vi "信号光谱9 - BN-BN.vi"() -> ()   [LabVIEW 2018]
uses:
  <vilib>/Utility/NIReport.llb/Report Type.ctl
  <vilib>/Utility/file.llb/Write Delimited Spreadsheet (DBL).vi
  <vilib>/Instr/_visa.llb/VISA Configure Serial Port (Instr).vi
  <vilib>/addons/_office/excel.llb/Excel Get Data ([str]).vi
  <vilib>/Utility/NIReport.llb/NI_report.lvclass
  <vilib>/Analysis/NI_AALBase.lvlib
  <vilib>/ptbypt/NI_PtbyPt.lvlib
  <vilib>/Utility/NIReport.llb/NI_ReportGenerationCore.lvlib
  <vilib>/addons/_office/NI_ReportGenerationToolkit.lvlib
  <vilib>/Utility/NIReport.llb/Excel/NI_Excel.lvclass
panel:
  out "数值":i32
  in  "停止预测":bool
  in  "误差值":dbl=0.5
  out "target angle":dbl
  out "图片地址 2":string
  out "图片地址 3":string
  out "原始峰值":dbl
  out "拟合峰值":dbl
  in  "角度倍乘系数":dbl=1.5
  out "结果展示":dbl[][](array[numeric])=[[37.33100777239877, 2672.955043835526, 29.54153292599307, 222755.0, 50.0], [37.36593979472361, 2672.656498058864, 30.113284142729572, 222833.0, 50.0], [38.96986225690859, 2673.3337152325566, 33.38805102415213, 222910.0, 75.0], [37.39946104045098, 2676.4005085744548, 31.215565446104666, 222948.0, 47.0], [35.862209164247574, 2671.7826876859012, 30.355582265151796, 223028.0, 47.0]]
  out "Δw2>C":bool=TRUE
  out "Δw1>C":bool=TRUE
  out "θi":dbl
  in  "w0":dbl format="%#_13g"
  in  "C=w-w0":dbl=180.0 format="%#_13g"
  in  "上升下降沿/s":dbl format="%.2p"
  in  "延时/s":dbl format="%.2p"
  in  "占空比/%":dbl=3.0 format="%.2p"
  in  "高电平/V":dbl=4.0 format="%.2p"
  in  "频率/Hz":dbl=6000.0 format="%.3p"
  in  "低电平/V":dbl min=0.0 max=5.0 format="%.2p"
  in  "Enable":bool
  in  "上升下降沿":i32(ring)=1 items=["上升沿", "下降沿"]
  in  "输出信号波形":u16(ring) items=["Pulse"]
  out "Output":bool
  in  "VISA 信号发生器":refnum<visa-resource-name>="USB0::0x1AB1::0x0641::DG4E192200870::INSTR"
  out "Output 2":bool
  in  "Enable 2":bool
  in  "上升下降沿/s 2":dbl format="%.2p"
  in  "延时/s 2":dbl format="%.2p"
  in  "占空比/% 2":dbl=3.0 format="%.2p"
  in  "高电平/V 2":dbl=0.002 format="%.2p"
  in  "频率/Hz 2":dbl=6000.0 format="%.3p"
  in  "低电平/V 2":dbl min=0.0 max=5.0 format="%.2p"
  in  "上升下降沿 2":i32(ring)=1 items=["上升沿", "下降沿"]
  in  "输出信号波形 2":u16(ring) items=["Pulse"]
  in  "终止测量":bool
  in  "测量次数":i32=1
  out "best fit":cluster{"Y":dbl[], "Y":dbl[]}[](graph)
  in  "拟合终点":i32=850
  in  "拟合起点":i32=200
  out "current angle":dbl
  out "图片地址":string
  in  "开光时间/ms":u32=50
  out "最终存储路径 2":path
  out "照明光error out":errorcluster
  in  "照明光":bool
  in  "stop bits (10: 1 bit)":u16(ring)=10 items=["1.0"=10, "1.5"=15, "2.0"=20]
  in  "parity (0:none)":enum16{"None", "Odd", "Even", "Mark", "Space"}(ring)
  in  "data bits (8)":u16=8 min=5 max=8 step=1
  in  "baud rate":u32=9600 caption="baud rate (115200)" min=9600 max=115200
  in  "照明光VISA":refnum<visa-resource-name>="COM12"
  out "正在测量":bool
  in  "滤波阈值":dbl=3000.0 format="%#_13g"
  out "范围内？":bool[](array[boolean])
  out "w":dbl
  out "xc":dbl
  out "拟合参数":dbl[](array[numeric])
  out "最终存储路径":path
  in  "停止程序":bool
  out "configure error out":errorcluster
  in  "设置参数":bool
  out "output control error  4":errorcluster
  in  "低电平持续输出":bool
  out "output control error  5":errorcluster
  out "output control error":errorcluster
  in  "开始测量":bool
  in  "channel输出口":i32(ring) items=["Channel 1", "Channel 2"]
  out "output control error":errorcluster
  out "Spectrum":cluster{"Y":dbl[], "Y":dbl[]}[](graph)
  out "波长范围":dbl[](array[numeric])
  in  "?":enum32{"IHR 550", "CCD"}(tab)
  in  "Move To\nTarget Positions":bool
  out "Current UniqueID":string="Mono4"
  in  "Mono ID":string(combo)="Mono1"
  in  "Connect":bool
  out "Initialized JY":bool=TRUE
  in  "Force\nInitialization":bool
  in  "Target Grating":string(combo)="2"
  out "Current Description":string="1" caption="Description"
  out "Grating Index":i32=1
  out "Current Grating":dbl=1200.0
  out "Units":string="nm"
  out "Current WL":dbl=897.9988
  out "Exit Mirror\nPosition":i32(ring)=2 items=["EntranceMirror", "ExitMirror", "Front", "Side"]
  out "Entrance Mirror\nPosition":i32(ring)=2 items=["EntranceMirror", "ExitMirror", "Front", "Side"]
  out "Units 2":string="mm"
  out "Front Entrance":dbl
  in  "Target WL":dbl=516.0
  in  "Exit Mirror":u16(ring)=3 caption="Target Position Exit Mirror" items=["Front"=2, "Side"=3]
  in  "Entrance Mirror":u16(ring)=2 caption="Target Position\nEntrance Mirror" items=["Front"=2, "Side"=3]
  in  "Target\nFront Entrance":dbl=2.0
  in  "Commande tab":T1(tab)
  in  "Area Number to Display":i32
  in  "Reformat":bool
  in  "GAIN":u16(ring)=2 caption="Device Name" items=["High Light", "Best Dynamic Range", "High Sensitivity"]
  in  "ADC":u16(ring) caption="Device Name" items=["20 kHz       ", " 1 MHz       ", " 1 MHz Ultra "]
  in  "Number of Areas :":u16=1 min=1 step=1
  in  "Integration time (ms) :":i16=10000
  out "Uniques ID":u16(ring) items=["CCD1", "CCD2"]
  in  "Device Name":u16(ring) items=["Synapse CCD (Lateral)", "Synapse_IGA (Axial)"]
  in  "Signal type :":enum16{"TTL Rising Edge", "TTL Falling Edge"}(ring)=enum."TTL Falling Edge"
  in  "Trigger Type :":u16(ring) items=["On Start"=1, "Per Acquisition"=2]
  in  "trigSigTypeString":string
  in  "trigEventString":string
  in  "Enable InputTriggers :":bool
  in  "Number of Cleans":i32=1
  in  "MultiAcqShutterMode":i32(ring)=3 items=["Open For All Spectra"=1, "Open for Each Spectrum"=3]
  in  "Accumulations:":u16=10 min=1 step=1
  in  "Multi Accumulation mode:":bool
  out "Y Pixels:":i32=256
  out "DataSize":i32=1024
  out "X Pixels:":i32=1024
  out "Firmware\nVersion":string="V1.20 CCD_4000"
  out "initialized ?":bool=TRUE
  in  "Continuous":bool
  in  "CCD Busy":bool
  out "indicator":string="Ready !"
  in  "initialize":bool
  in  "ShutterOpen":bool=TRUE caption="Shutter enable"
  in  "Acquire":bool
  in  "Temperature":bool
  in  "Setup":bool
  out "Acq Time(ms)":u32=3401
  in  "Save Backlight":bool
  in  "cut backlight":bool
  out "backlight":bool=TRUE
  in  "是否拟合":bool
  in  "是否保存":bool
  in  "Close":bool=TRUE
  out "JYCCDLib.IJYCCDReqd":refnum<k7>
  out "areas :":i32[][](array[numeric])=[[1], [1], [1], [1024], [256], [1], [256]]
  in  "Constante de condition\n(Voir l'aide contextuelle)":bool
  out "temp graph":dbl(graph)=-134.538067
  out "ADC Number":i32[](array[numeric])=[0, 1, 2, 3, 4]
  out "Gain Number":i32[](array[numeric])=[10, 11, 12, 13, 8, 2]
  out "trigAddress":i32
  out "Data":i32[][](graph)
  out "error out":errorcluster
  out "Gratings":dbl[](array[numeric])=[1200.0, 300.0]
  out "Backlight":i32[][](graph)
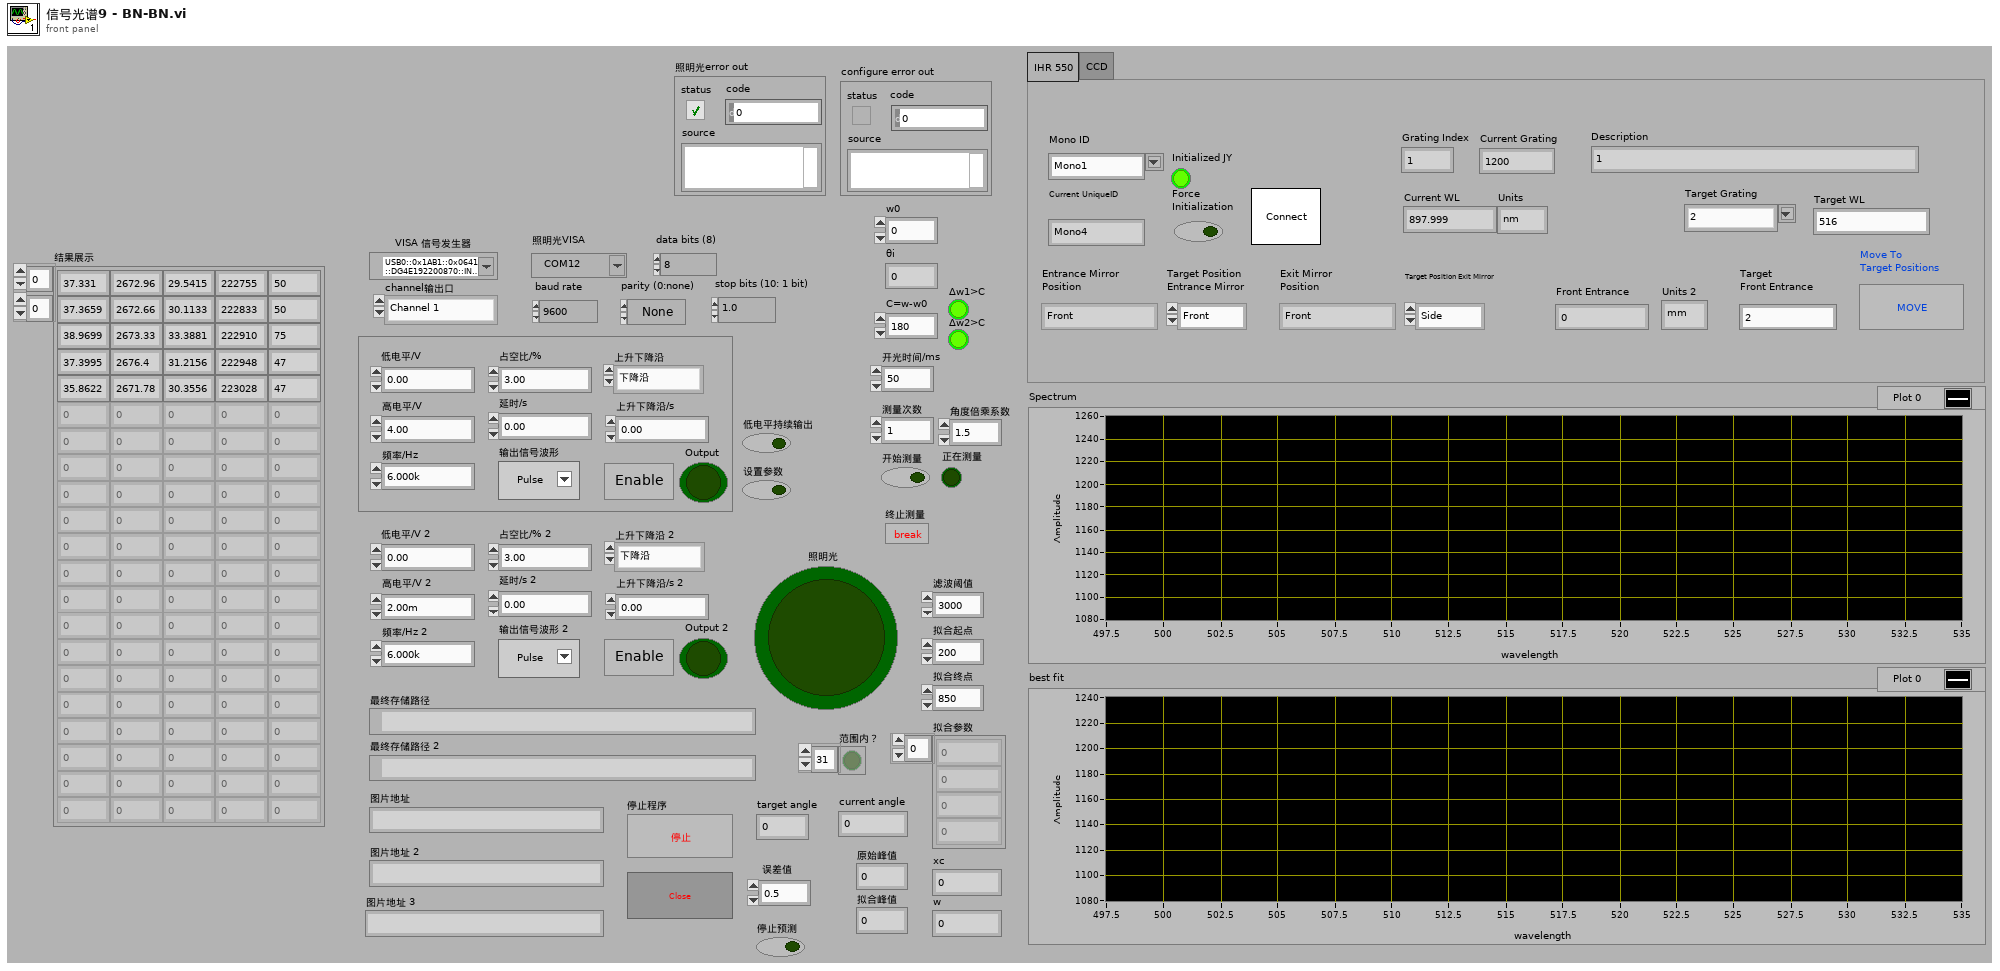
[diagram p1: front panel]
types:
  T1 = enum32{"Settings", "Trigger In", "Multi-Accu.", "Infos"}
  T2 = enum8{"Enabled", "Disabled", "Disabled and Grayed Out"}
  T3 = enum16{"maximized", "minimized", "normal", "no change"}
  T4 = typedef "NI_ReportGenerationCore.lvlib/Report Type.ctl" = enum16{"HTML", "Word", "Excel"}
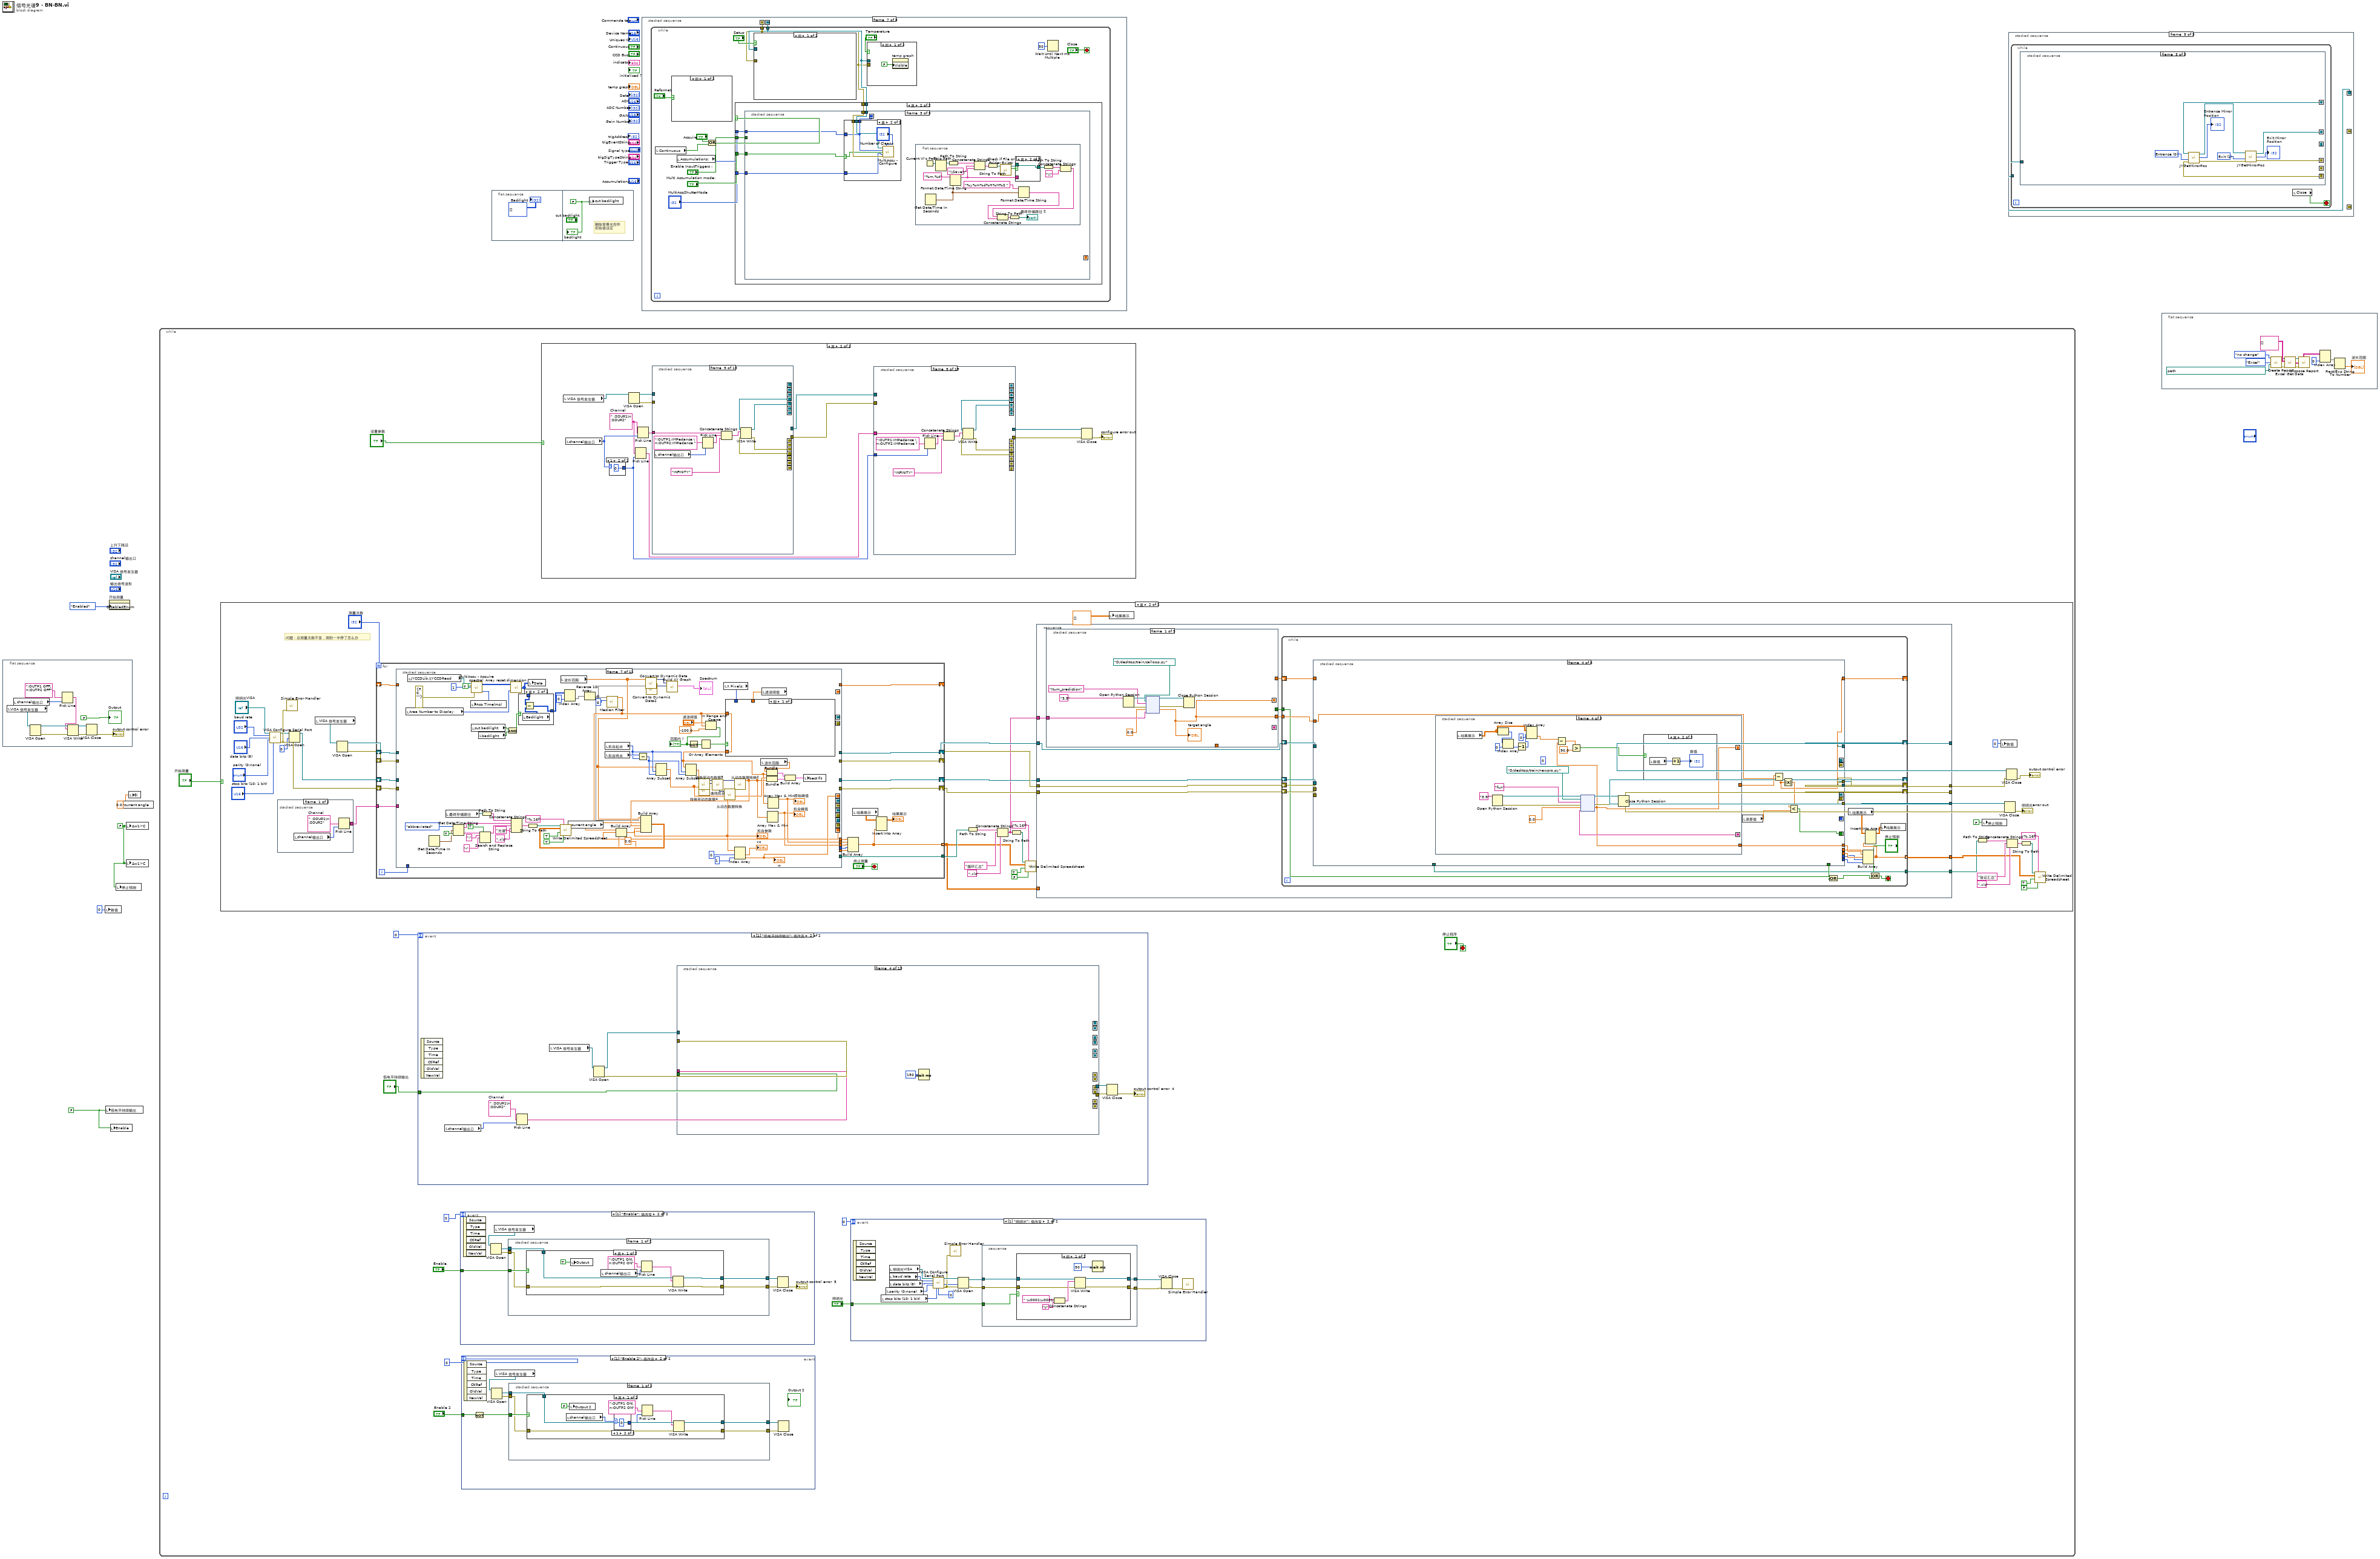
[diagram p0: block diagram]
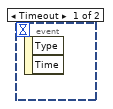
[diagram p2: hidden frame]
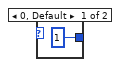
[diagram p3: hidden frame]
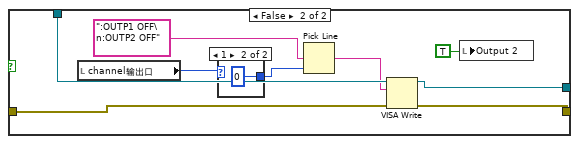
[diagram p4: hidden frame]
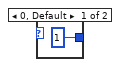
[diagram p5: hidden frame]
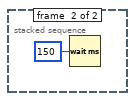
[diagram p6: hidden frame]
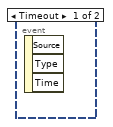
[diagram p7: hidden frame]
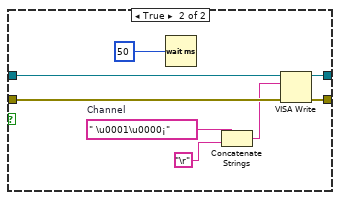
[diagram p8: hidden frame]
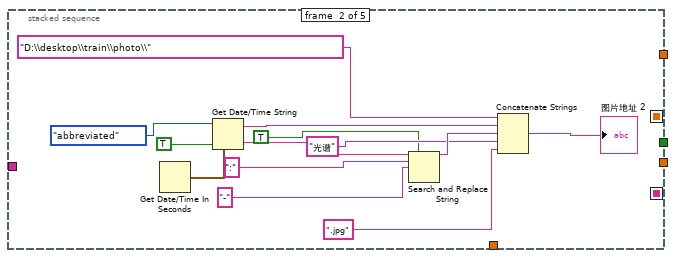
[diagram p10: hidden frame]
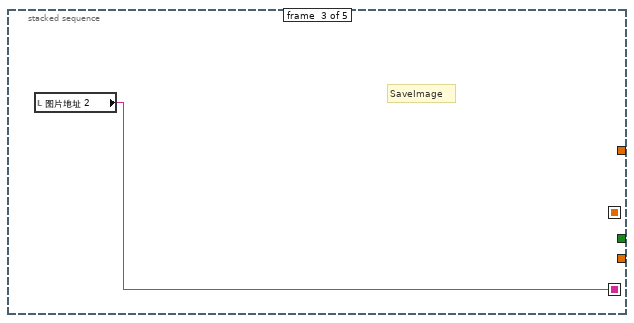
[diagram p11: hidden frame]
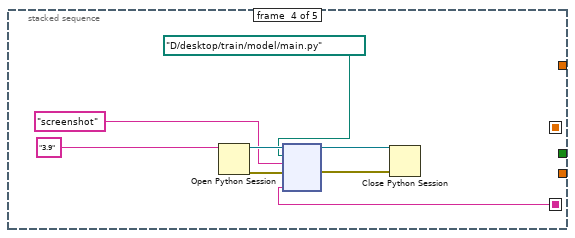
[diagram p12: hidden frame]
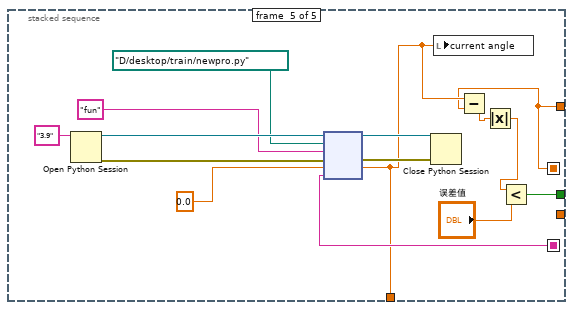
[diagram p13: hidden frame]
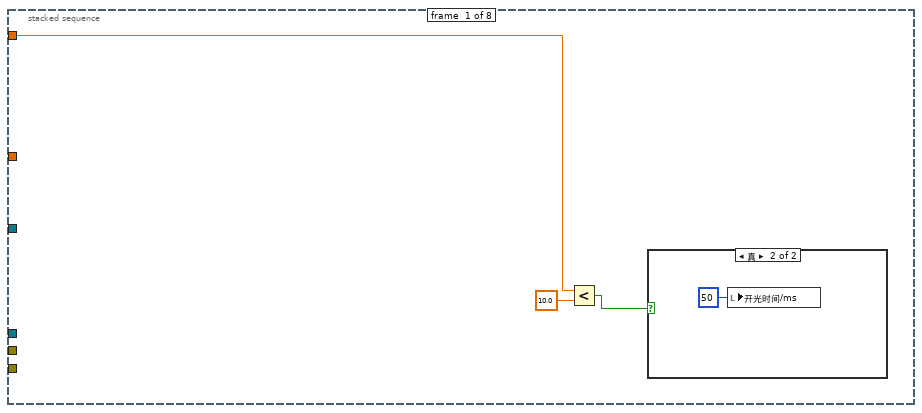
[diagram p14: hidden frame]
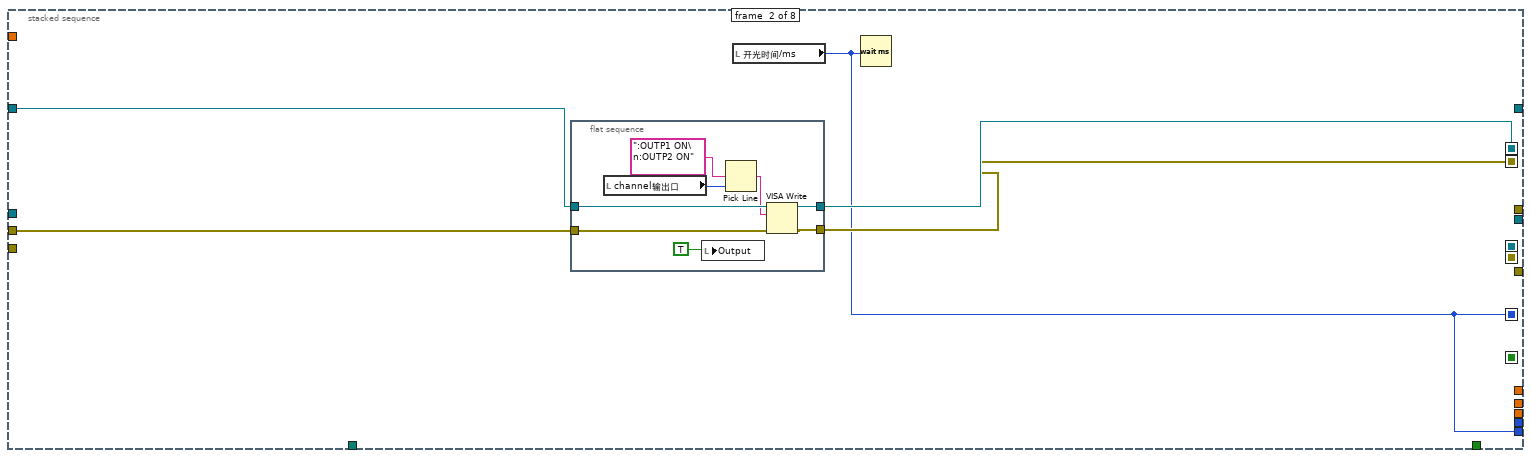
[diagram p16: hidden frame]
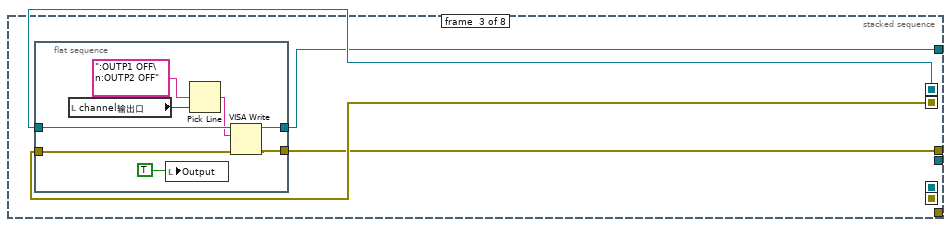
[diagram p17: hidden frame]
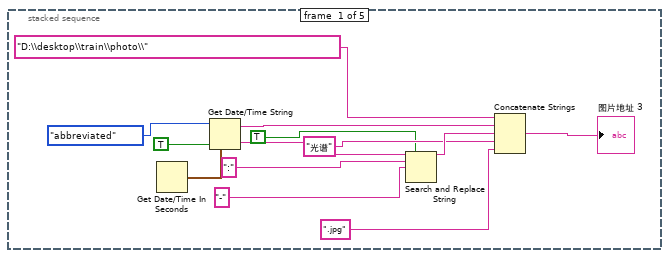
[diagram p18: hidden frame]
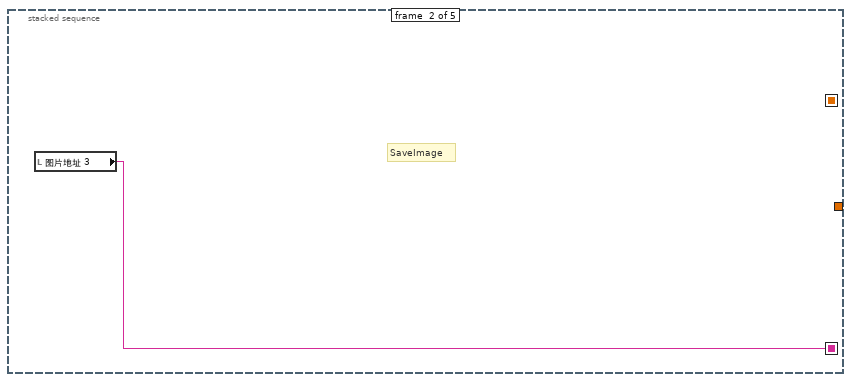
[diagram p19: hidden frame]
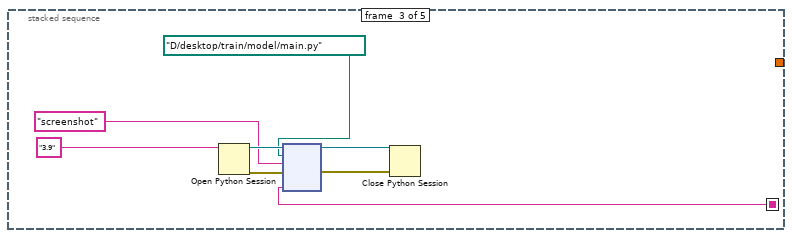
[diagram p20: hidden frame]
diagram:
  w2 = FALSE ("Δw1>C")
  w3 = 0.0 ("angle")
  w4 = FALSE
  n1 = flat-sequence {
    frame #0 {
      n2 = local read "VISA 信号发生器"() -> (w9:refnum<visa-resource-name>)
      n3 = local read "channel输出口"() -> (w7:i32)
      n4 = VISA Open(VISA resource name=w9) -> (VISA resource name=w15:refnum<visa-resource-name>, error out=w14:errorcluster)  [unwired: 4 in]
      n5 = Pick Line(multi-line string=":OUTP1 OFF\n:OUTP2 OFF" ("write buffer"), line index=w7) -> (output string=w6:string)  [unwired: 1 in]
      n6 = VISA Write(VISA resource name=w15, write buffer=w6, error in (no error)=w14) -> (VISA resource name out=w12:refnum<visa-resource-name>, error out=w11:errorcluster)  [unwired: 1 out]
      n7 = VISA Close(VISA resource name=w12, error in (no error)=w11) -> (error out=→"output control error":errorcluster)
      "Output" <- FALSE ("布尔")
    }
  }
  n8 = local write "数值"(0 ("数值")) -> ()
  n9 = local write "低电平持续输出"(w4) -> ()
  n10 = property on="开始测量" class="Bool"("DisabledEnum"=T2."Enabled" ("禁用")) -> ()  [unwired: 2 in, 2 out]
  n11 = local write "Enable"(w4) -> ()
  n12 = local write "停止预测"(w2) -> ()
  n13 = local write "current angle"(w3) -> ()
  n14 = local write "Δw1>C"(w2) -> ()
  n15 = local write "Δw1>C"(w2) -> ()
  n16 = local write "θi"(w3) -> ()
  n17 = while {
    stop <- "停止程序" stop-if-true
    n18 = case shown="真" "开始测量" {
      frame False {
      }
      frame True {
        # "问题：总测量次数不变，测到一半停了怎么办"
        n19 = call-poly "VISA Configure Serial Port"("VISA resource name"="照明光VISA", "baud rate (9600)"="baud rate", "data bits (8)"="data bits (8)", "parity (0:none)"="parity (0:none)", "stop bits (10: 1 bit)"="stop bits (10: 1 bit)") -> ("VISA resource name out"=w139:refnum<visa-resource-name>, "error out"=w140:errorcluster)  [unwired: 9 in]
        n20 = stacked-sequence {
          tunnel: [w437 _] -> w141
          frame #0 {
            w438 = " :SOUR1\n :SOUR2"  # Channel
            n21 = local read "channel输出口"() -> (w439:i32)
            n22 = Pick Line(multi-line string=w438, line index=w439) -> (output string=w437:string)  [unwired: 1 in]
          }
          frame #1 {
            w440 = FALSE ("Δw1>C")
            n23 = local write "Δw1>C"(w440) -> ()
            n24 = local write "Δw2>C"(w440) -> ()
          }
        }
        n25 = call <vilib>:"Simple Error Handler.vi"("error in (no error)"=w140) -> ()  [unwired: 4 in, 5 out]
        n26 = VISA Open(access mode=0, error in (no error)=w140, VISA resource name=w139) -> (VISA resource name=w132:refnum<visa-resource-name>, error out=w131:errorcluster)  [unwired: 2 in]
        n27 = local read "VISA 信号发生器"() -> (w144:refnum<visa-resource-name>)
        n28 = VISA Open(VISA resource name=w144) -> (VISA resource name=w143:refnum<visa-resource-name>, error out=w142:errorcluster)  [unwired: 4 in]
        n29 = for {
          N: "测量次数" -> [_]
          tunnel: w141 -> [w460]
          shift-right: [w456] -> w119
          shift-left: w143 -> [w462]
          shift-right: [w455] -> w118
          shift-left: w142 -> [w461]
          shift-right: [w454] -> w113
          shift-left: w132 -> [w459]
          shift-right: [w453] -> w112
          shift-left: w131 -> [w458]
          tunnel: [w443] -> w120 mode=indexing
          shift-right: [w448] -> _
          shift-left: _ -> [w447]
          tunnel: [w444] -> w122
          i -> [w446]
          stop <- "终止测量" stop-if-true
          n30 = stacked-sequence {
            seq-local: [w469 _ _ _ _ _ _ _ _ _ _ _] -> [_ w489 _ _ _ _ _ _ _ _ _ _]
            seq-local: [w468 _ _ _ _ _ _ _ _ _ _ _] -> [_ w488 _ _ _ _ _ _ _ _ _ _]
            seq-local: [_ _ _ _ _ w574 _ _ _ _ _ _] -> [_ _ _ _ _ _ _ _ w692 _ _ _]
            seq-local: [_ _ _ _ _ w573 _ _ _ _ _ _] -> [_ _ _ _ _ _ _ _ w695 _ _ _]
            seq-local: [_ w487 _ _ _ _ _ _ _ _ _ _] -> [_ _ _ _ w560 _ _ _ _ _ _ _]
            seq-local: [_ w486 _ _ _ _ _ _ _ _ _ _] -> [_ _ _ _ w559 _ _ _ _ _ _ _]
            seq-local: [_ _ _ _ w558 _ _ _ _ _ _ _] -> [_ _ _ _ _ _ _ w678 _ _ _ _]
            seq-local: [_ _ _ _ w557 _ _ _ _ _ _ _] -> [_ _ _ _ _ _ _ w677 _ _ _ _]
            seq-local: [_ _ w498 _ _ _ _ _ _ _ _ _] -> [_ _ _ _ _ _ _ _ _ _ w704 _]
            seq-local: [_ _ _ _ _ _ w589 _ _ _ _ _] -> [_ _ _ _ _ _ _ _ _ _ w699 _]
            seq-local: [w463 _ _ _ _ _ _ _ _ _ _ _] -> [_ _ _ _ _ _ w587 _ _ _ _ _]
            tunnel: w462 -> [w471 _ _ _ _ _ _ _ _ _ _ _]
            tunnel: w461 -> [w470 _ _ _ _ _ _ _ _ _ _ _]
            tunnel: [_ _ _ _ _ _ _ w676 _ _ _ _] -> w456
            tunnel: [_ _ _ _ _ _ _ w675 _ _ _ _] -> w455
            tunnel: w460 -> [_ _ _ _ _ _ _ _ _ _ _ _]
            tunnel: w459 -> [_ _ _ _ _ w577 _ _ _ _ _ _]
            tunnel: w458 -> [_ _ _ _ _ w576 _ _ _ _ _ _]
            tunnel: [_ _ _ _ _ _ _ _ w694 _ _ _] -> w454
            tunnel: [_ _ _ _ _ _ _ _ w693 _ _ _] -> w453
            tunnel: [_ _ w498 _ _ _ _ _ _ _ _ _] -> w452
            tunnel: [_ _ _ _ _ _ w584 _ _ _ _ _] -> w451
            tunnel: [_ _ _ _ _ _ w583 _ _ _ _ _] -> w450
            tunnel: [_ _ _ w532 _ _ _ _ _ _ _ _] -> w449
            tunnel: [w463 _ _ _ _ _ _ _ _ _ _ _] -> w445
            tunnel: [_ _ w498 _ _ _ _ _ _ _ _ _] -> w448
            tunnel: w447 -> [_ _ _ _ _ _ _ _ _ _ w703 _]
            tunnel: w446 -> [_ _ _ _ _ _ _ _ _ _ w701 _]
            tunnel: [_ _ _ w531 _ _ _ _ _ _ _ _] -> w444
            frame #0 {
              n31 = Wait Until Next ms Multiple(millisecond multiple=u32 1 ("毫秒倍数")) -> ()  [unwired: 1 out]
              n32 = flat-sequence {
                tunnel: w471 -> [w485]
                tunnel: w470 -> [w484]
                tunnel: [w479] -> w469
                tunnel: [w478] -> w468
                frame #0 {
                  n33 = local read "channel输出口"() -> (w481:i32)
                  n34 = local write "Output"(TRUE ("布尔")) -> ()
                  n35 = Pick Line(multi-line string=":OUTP1 ON\n:OUTP2 ON" ("write buffer"), line index=w481) -> (output string=w480:string)  [unwired: 1 in]
                  n36 = VISA Write(VISA resource name=w485, write buffer=w480, error in (no error)=w484) -> (VISA resource name out=w479:refnum<visa-resource-name>, error out=w478:errorcluster)  [unwired: 1 out]
                }
              }
              n37 = local read "Δw1>C"() -> (w465:bool)
              n38 = local read "Δw2>C"() -> (w466:bool)
              n39 = And(x=w465, y=w466) -> (x .and. y?=w464:bool)
              n40 = case shown="真" w464 {
                tunnel: [w474 w475] -> w463
                tunnel: "开光时间/ms" -> [w474 w477]
                frame False {
                }
                frame True {
                  n41 = Divide(x=w477, y=u32 4) -> (x/y=w475:dbl)
                }
              }
              n42 = Wait (ms)(milliseconds to wait=w463) -> ()  [unwired: 1 out]
              "正在测量" <- TRUE
            }
            frame #1 {
              n43 = flat-sequence {
                tunnel: w489 -> [w497]
                tunnel: w488 -> [w496]
                tunnel: [w491] -> w487
                tunnel: [w490] -> w486
                frame #0 {
                  n44 = local read "channel输出口"() -> (w493:i32)
                  n45 = local write "Output"(FALSE ("布尔")) -> ()
                  n46 = Pick Line(multi-line string=":OUTP1 OFF\n:OUTP2 OFF" ("write buffer"), line index=w493) -> (output string=w492:string)  [unwired: 1 in]
                  n47 = VISA Write(VISA resource name=w497, write buffer=w492, error in (no error)=w496) -> (VISA resource name out=w491:refnum<visa-resource-name>, error out=w490:errorcluster)  [unwired: 1 out]
                }
              }
            }
            frame #2 {
              n48 = stacked-sequence {
                seq-local: [_ w512 _ _] -> [_ _ w513 w522]
                tunnel: [_ _ _ w521] -> w498
                frame #0 {
                  n49 = Get Date/Time In Seconds() -> (seconds since 1Jan1904=w508:timestamp)
                  n50 = Get Date/Time String(date format (0)=enum16{"short", "long", "abbreviated"}."abbreviated" ("日期格式(0)"), seconds (now)=w508, want seconds? (F)=TRUE ("需要秒？(F)")) -> (date string=w511:string, time string=w509:string)
                  n51 = Search and Replace String(replace all?=TRUE ("替换全部？(F)"), input string=w509, search string=":" ("搜索字符串"), replace string="-" ("替换字符串(\"\")")) -> (result string=w510:string)  [unwired: 4 in, 3 out]
                  n52 = Concatenate Strings("D:\\desktop\\train\\photo\\", w511, w510, "光谱" ("字符串"), ".jpg" ("字符串")) -> (→"图片地址":string)
                }
                frame #1 {
                  # "SaveImage"
                  n53 = local read "图片地址"() -> (w512:string)
                }
                frame #2 {
                  n54 = Open Python Session(python version="3.9" ("Python version")) -> (session out=w520:refnum<k35>, error out=w518:errorcluster)  [unwired: 2 in]
                  n55 = node(w520, path "D:/desktop/train/model/main.py" ("module path"), "screenshot" ("function name"), w518, w513) -> (w519:refnum<k35>, w517:errorcluster)  [unwired: 3 in, 2 out]
                  n56 = Close Python Session(session in=w519, error in=w517) -> ()  [unwired: 1 out]
                }
                frame #3 {
                  n57 = Open Python Session(python version="3.9" ("Python version")) -> (session out=w529:refnum<k35>, error out=w527:errorcluster)  [unwired: 2 in]
                  n58 = node(w529, path "D:/desktop/train/newpro.py" ("module path"), "fun" ("function name"), w527, 0.0, w522) -> (w528:refnum<k35>, w526:errorcluster, w521:dbl)  [unwired: 1 in, 2 out]
                  "current angle" <- w521
                  n59 = Close Python Session(session in=w528, error in=w526) -> ()  [unwired: 1 out]
                }
              }
            }
            frame #3 {
              n60 = Current VI's Path() -> (path=w541:path)
              n61 = Get Date/Time In Seconds() -> (seconds since 1Jan1904=w534:timestamp)
              n62 = Strip Path(path=w541) -> (stripped path=w542:path)  [unwired: 1 out]
              n63 = Path To String(path=w542) -> (string=w543:string)
              n64 = Format Date/Time String(time format string (%c)="%m-%d" ("时间格式字符串(%c)"), seconds (now)=w534) -> (date/time string=w549:string)  [unwired: 1 in]
              n65 = Concatenate Strings(w543, "\\Save\\" ("字符串"), w549) -> (w544:string)
              n66 = String To Path(string=w544) -> (path=w545:path)
              n67 = call <vilib>:"Check if File or Folder Exists.vi"("path"=w545) -> ("file or folder exists?"=w546:bool, "dup path"=w548:path)  [unwired: 8 in, 1 out]
              n68 = case shown="真" w546 {
                tunnel: [w555 w556] -> w547
                tunnel: w548 -> [w554 w556]
                tunnel: w549 -> [w553 _]
                frame False {
                  n69 = Create Folder(prompt (Create Folder)=w553, path (use dialog)=w554) -> (created path=w555:path)  [unwired: 1 in, 2 out]
                }
                frame True {
                }
              }
              n70 = Format Date/Time String(time format string (%c)="%y%m%d%H%M%S" ("时间格式字符串(%c)"), seconds (now)=w534) -> (date/time string=w552:string)  [unwired: 1 in]
              n71 = Path To String(path=w547) -> (string=w550:string)
              n72 = Concatenate Strings(w550, "\\" ("字符串")) -> (w551:string)
              n73 = Format Date/Time String(time format string (%c)="%H%M%S" ("时间格式字符串(%c)"), seconds (now)=w534) -> (date/time string=w533:string)  [unwired: 1 in]
              n74 = Concatenate Strings(w551, w552) -> (w540:string)
              n75 = String To Path(string=w540) -> (path=w531:path)
              "最终存储路径" <- w531
              n76 = Decimal String To Number(string=w533) -> (number=w532:i32)  [unwired: 2 in, 1 out]
            }
            frame #4 {
              n77 = flat-sequence {
                tunnel: w560 -> [w569]
                tunnel: w559 -> [w568]
                tunnel: [w564] -> w558
                tunnel: [w563] -> w557
                frame #0 {
                  n78 = local read "channel输出口"() -> (w562:i32)
                  n79 = case shown="1" w562 {
                    tunnel: [1 0] -> w561
                    frame 0, Default {
                    }
                    frame 1 {
                    }
                  }
                  n80 = local write "Output 2"(FALSE ("布尔")) -> ()
                  n81 = Pick Line(multi-line string=":OUTP1 OFF\n:OUTP2 OFF" ("write buffer"), line index=w561) -> (output string=w565:string)  [unwired: 1 in]
                  n82 = VISA Write(VISA resource name=w569, write buffer=w565, error in (no error)=w568) -> (VISA resource name out=w564:refnum<visa-resource-name>, error out=w563:errorcluster)  [unwired: 1 out]
                }
              }
            }
            frame #5 {
              w572 = " \u0001\u0001¢"  # Channel
              n83 = Wait (ms)(milliseconds to wait=500) -> ()  [unwired: 1 out]
              n84 = Concatenate Strings(w572, "\r") -> (w578:string)
              n85 = local write "照明光"(FALSE ("照明光")) -> ()
              n86 = VISA Write(VISA resource name=w577, write buffer=w578, error in (no error)=w576) -> (VISA resource name out=w574:refnum<visa-resource-name>, error out=w573:errorcluster)  [unwired: 1 out]
            }
            frame #6 {
              n87 = local read "Area Number to Display"() -> (w628:i32)
              n88 = local read "JYCCDLib.IJYCCDReqd"() -> (w624:refnum<k7>)
              n89 = Get Date/Time In Seconds() -> (seconds since 1Jan1904=w637:timestamp)
              n90 = local read "最终存储路径"() -> (w651:path)
              n91 = Get Date/Time String(date format (0)=enum16{"short", "long", "abbreviated"}."abbreviated" ("日期格式(0)"), seconds (now)=w637, want seconds? (F)=TRUE ("需要秒？(F)")) -> (date string=w645:string, time string=w640:string)
              n92 = call "MultiAccu - Acquire spectral.vi"("error in"=errorcluster {"status"=FALSE, "code"=0, "source"=""}, "Accumulations:"=u16 1, "ShutterOpen"=TRUE, "JYCCDLib.IJYCCDReqd"=w624) -> ("Acq Time(ms)"=w630:u32, "Array Out"=w629:i32[][][])  [unwired: 1 out]
              n93 = local write "Acq Time(ms)"(w630) -> ()
              n94 = local read "cut backlight"() -> (w612:bool)
              n95 = local read "backlight"() -> (w610:bool)
              n96 = Search and Replace String(replace all?=TRUE ("替换全部？(F)"), input string=w640, search string=":" ("搜索字符串"), replace string="-" ("替换字符串(\"\")")) -> (result string=w644:string)  [unwired: 4 in, 3 out]
              n97 = Path To String(path=w651) -> (string=w634:string)
              n98 = And(x=w612, y=w610) -> (x .and. y?=w611:bool)
              n99 = call "Array reset dimension.vi"("Area Number"=w628, "Array In"=w629) -> ("Array Out"=w614:i32[][])
              n100 = Concatenate Strings(w634, w645, w644, "光谱" ("字符串"), ".xls" ("字符串")) -> (w649:string)
              n101 = case shown="真" w611 {
                tunnel: [w671 w673] -> w613
                tunnel: w614 -> [w671 w672]
                frame False {
                }
                frame True {
                  n102 = local read "Backlight"() -> (w674:i32[][])
                  n103 = Subtract(x=w672, y=w674) -> (x-y=w673:i32[][])
                }
              }
              n104 = String To Path(string=w649) -> (path=w650:path)
              n105 = local write "Data"(w614) -> ()
              n106 = local read "波长范围"() -> (w582:dbl[])
              n107 = Index Array(array=w613, index (row)=0 ("索引 (行)")) -> (element=w652:i32[])  [unwired: 1 in]
              n108 = local read "current angle"() -> (w593:dbl)
              n109 = Reverse 1D Array(array=w652) -> (reversed array=w581:i32[])
              n110 = local read "拟合起点"() -> (w600:i32)
              n111 = local read "拟合终点"() -> (w602:i32)
              n112 = call <vilib>:"Median Filter.vi"("left rank"=6, "X"=w581) -> ("Filtered X"=w591:dbl[])  [unwired: 8 in, 1 out]
              n113 = Build Array(w593, w587, 0.0 ("元素")) -> (w592:dbl[])
              n114 = Subtract(x=w602, y=w600) -> (x-y=w599:i32)
              n115 = call "Convert to Dynamic Data"("Array"=w582) -> ("Dynamic Data Type"=w621:dynamicdata)  [unwired: 3 in]
              n116 = call "Convert to Dynamic Data2"("Array"=w581) -> ("Dynamic Data Type"=w620:dynamicdata)  [unwired: 3 in]
              n117 = Array Subset(array=w582, index=w600, length=w599) -> (w598:dbl[])
              n118 = call "Build XY Graph"("Y Input"=w620, "X Input"=w621) -> ("XY Graph"=→"Spectrum":cluster{"Y":dbl[], "Y":dbl[]}[])  [unwired: 8 in, 1 out]
              n119 = call "转换至动态数据4"("Array"=w598) -> ("Dynamic Data Type"=w618:dynamicdata)  [unwired: 3 in]
              n120 = In Range and Coerce(upper limit="滤波阈值", x=w591, lower limit=-100.0) -> (In Range?=w605:bool[])  [unwired: 1 out]
              "范围内？" <- w605
              n121 = Not(x=w605) -> (.not. x?=w604:bool[])
              n122 = Or Array Elements(Boolean array=w604) -> (logical OR=w607:bool)
              n123 = local read "X Pixels:"() -> (w606:i32)
              n124 = local read "波长范围"() -> (w594:dbl[])
              n125 = local read "滤波阈值"() -> (w603:dbl)
              n126 = case shown="假" w607 {
                tunnel: w606 -> [_ w658]
                tunnel: w591 -> [w654 w657]
                tunnel: [w654 w656] -> w585
                tunnel: w603 -> [_ w655]
                frame False {
                }
                frame True {
                  n127 = for {
                    N: w658 -> [_]
                    tunnel: w657 -> [w662] mode=indexing
                    tunnel: [w661] -> w656 mode=indexing
                    shift-right: [w661] -> _
                    shift-left: _ -> [w660]
                    tunnel: w655 -> [w659]
                    n128 = Greater?(x=w662, y=w659) -> (0:w664:bool)
                    n129 = Less?(x=w662, y=-100.0) -> (x < y?=w665:bool)
                    n130 = Or(x=w664, y=w665) -> (x .or. y?=w663:bool)
                    n131 = case shown="真" w663 {
                      tunnel: w662 -> [w667 _]
                      tunnel: [w667 w669] -> w661
                      tunnel: w660 -> [_ w670]
                      frame False {
                      }
                      frame True {
                        n132 = call <vilib>:"Median Filter PtByPt.vi"("rank"=5, "x"=w670) -> ("Filtered x"=w669:dbl)  [unwired: 2 in, 1 out]
                      }
                    }
                  }
                }
              }
              n133 = Array Subset(array=w585, index=w600, length=w599) -> (w601:dbl[])
              n134 = call "转换至动态数据3"("Array"=w601) -> ("Dynamic Data Type"=w619:dynamicdata)  [unwired: 3 in]
              n135 = call "曲线拟合"("Locations"=w618, "Signals"=w619) -> ("best fit"=w623:dynamicdata, "non-linear coefficients"=w622:dynamicdata)  [unwired: 5 in, 3 out]
              n136 = call "从动态数据转换"("Dynamic Data Type"=w622) -> ("Array"=w615:dbl[])  [unwired: 3 in]
              "拟合参数" <- w615
              n137 = call "从动态数据转换2"("Dynamic Data Type"=w623) -> ("Array"=w586:dbl[])  [unwired: 3 in]
              n138 = Build Array(w582, w581, w591, w586, w615, w592) -> (w653:dbl[][])
              n139 = call-poly <vilib>:"Write Delimited Spreadsheet.vi"("file path (dialog if empty)"=w650, "format (%.3f)"="%.16f", "2D data"=w653, "append to file? (new file:F)"=TRUE ("append to file? (F)"), "transpose? (no:F)"=TRUE ("transpose? (F)")) -> ()  [unwired: 9 in, 2 out]
              n140 = Index Array(array=w615, index #1=0 ("索引"), index #2=1 ("索引")) -> (element #1=→"xc":dbl, element #2=w589:dbl)
              "w" <- w589
              n141 = Bundle("波长范围"=w594, "Filtered X"=w585) -> (w597:cluster{"波长范围 ":dbl[], "Filtered X":dbl[]})  [unwired: 1 in]
              n142 = Bundle(w598, "Array"=w586) -> (w596:cluster{dbl[], "Array":dbl[]})  [unwired: 1 in]
              n143 = Array Max & Min(array=w586) -> (max value=w583:dbl)  [unwired: 3 out]
              "拟合峰值" <- w583
              n144 = Array Max & Min(array=w585) -> (max value=w584:dbl)  [unwired: 3 out]
              "原始峰值" <- w584
              n145 = Build Array(w597, w596) -> (w595:cluster{"波长范围 ":dbl[], "Array":dbl[]}[])
              n146 = local write "best fit"(w595) -> ()
            }
            frame #7 {
              n147 = flat-sequence {
                tunnel: w678 -> [w687]
                tunnel: w677 -> [w686]
                tunnel: [w682] -> w676
                tunnel: [w681] -> w675
                frame #0 {
                  n148 = local read "channel输出口"() -> (w680:i32)
                  n149 = case shown="1" w680 {
                    tunnel: [1 0] -> w679
                    frame 0, Default {
                    }
                    frame 1 {
                    }
                  }
                  n150 = local write "Output 2"(TRUE ("布尔")) -> ()
                  n151 = Pick Line(multi-line string=":OUTP1 ON\n:OUTP2 ON" ("write buffer"), line index=w679) -> (output string=w683:string)  [unwired: 1 in]
                  n152 = VISA Write(VISA resource name=w687, write buffer=w683, error in (no error)=w686) -> (VISA resource name out=w682:refnum<visa-resource-name>, error out=w681:errorcluster)  [unwired: 1 out]
                }
              }
            }
            frame #8 {
              w690 = " \u0001\u0000¡"  # Channel
              n153 = Concatenate Strings(w690, "\r") -> (w696:string)
              n154 = VISA Write(VISA resource name=w692, write buffer=w696, error in (no error)=w695) -> (VISA resource name out=w694:refnum<visa-resource-name>, error out=w693:errorcluster)  [unwired: 1 out]
              n155 = local write "照明光"(TRUE ("照明光")) -> ()
            }
            frame #9 {
              n156 = Wait (ms)(milliseconds to wait=1200) -> ()  [unwired: 1 out]
            }
            frame #10 {
              n157 = Greater Or Equal?(x=w701, y=1) -> (x >= y?=w702:bool)
              n158 = case shown="真" w702 {
                tunnel: w704 -> [_ w710]
                tunnel: w703 -> [_ w711]
                tunnel: w699 -> [w705 w712]
                frame False {
                  n159 = local write "w0"(w705) -> ()
                }
                frame True {
                  n160 = local read "Δw1>C"() -> (w709:bool)
                  n161 = case shown="假" w709 {
                    tunnel: w712 -> [w731 w751]
                    tunnel: w711 -> [w721 _]
                    tunnel: w710 -> [w722 _]
                    frame False {
                      # "判断Δw突变位置并记录当前θ值"
                      # "根据θ变化速度改变开光时间"
                      n162 = local read "w0"() -> (w729:dbl)
                      n163 = Subtract(x=w722, y=w721) -> (x-y=w724:dbl)
                      n164 = local read "开光时间/ms"() -> (w727:u32)
                      n165 = Subtract(x=w729, y=w731) -> (x-y=w734:dbl)
                      n166 = Absolute Value(x=w724) -> (abs(x)=w726:dbl)
                      n167 = Absolute Value(x=w734) -> (abs(x)=w732:dbl)
                      n168 = Greater Or Equal?(x=w726, y=4.0) -> (x >= y?=w725:bool)
                      n169 = Greater Or Equal?(x=w732, y="C=w-w0") -> (x >= y?=w730:bool)
                      n170 = case shown="真" w730 {
                        tunnel: w721 -> [_ w749]
                        frame False {
                          w747 = FALSE ("Δw1>C")
                          n171 = local write "Δw1>C"(w747) -> ()
                          n172 = local write "Δw2>C"(w747) -> ()
                        }
                        frame True {
                          "θi" <- w749
                          "Δw1>C" <- TRUE ("布尔")
                        }
                      }
                      n173 = case shown="假" w725 {
                        tunnel: w726 -> [w739 _]
                        tunnel: w727 -> [w736 w746]
                        tunnel: [w735 w744] -> w728
                        frame False {
                          n174 = Less Or Equal?(x=w739, y=1.0) -> (x <= y?=w737:bool)
                          n175 = case shown="假" w737 {
                            tunnel: w736 -> [w740 w743]
                            tunnel: [w740 w742] -> w735
                            frame False {
                            }
                            frame True {
                              n176 = Multiply(x=w743, y="角度倍乘系数") -> (x*y=w742:dbl)
                            }
                          }
                        }
                        frame True {
                          n177 = Divide(x=w746, y=1.6) -> (x/y=w744:dbl)
                        }
                      }
                      n178 = local write "开光时间/ms"(w728) -> ()
                    }
                    frame True {
                      # "再次判断Δw，排除坏点影响"
                      n179 = local read "Δw2>C"() -> (w750:bool)
                      n180 = case shown="假" w750 {
                        tunnel: w751 -> [w756 _]
                        frame False {
                          n181 = local read "C=w-w0"() -> (w753:dbl)
                          n182 = local read "w0"() -> (w757:dbl)
                          n183 = Subtract(x=w757, y=w756) -> (x-y=w759:dbl)
                          n184 = Absolute Value(x=w759) -> (abs(x)=w758:dbl)
                          n185 = Add(x=w753, y=0.5) -> (x+y=w752:dbl)
                          n186 = Greater Or Equal?(x=w758, y=w752) -> (x >= y?=w755:bool)
                          n187 = case shown="真" w755 {
                            frame False {
                              n188 = local write "θi"(0.0 ("θi")) -> ()
                              n189 = local write "Δw1>C"(FALSE ("Δw1>C")) -> ()
                            }
                            frame True {
                              "Δw2>C" <- TRUE
                            }
                          }
                        }
                        frame True {
                        }
                      }
                    }
                  }
                  n190 = local read "Δw1>C"() -> (w707:bool)
                  n191 = local read "Δw2>C"() -> (w708:bool)
                  n192 = And(x=w707, y=w708) -> (x .and. y?=w706:bool)
                  n193 = case shown="真" w706 {
                    tunnel: w710 -> [_ w713]
                    frame False {
                    }
                    frame True {
                      # "4°后重置指示灯状态"
                      n194 = local read "θi"() -> (w717:dbl)
                      n195 = Subtract(x=w713, y=w717) -> (x-y=w718:dbl)
                      n196 = Absolute Value(x=w718) -> (abs(x)=w716:dbl)
                      n197 = Greater?(x=w716, y=4.0) -> (0:w714:bool)
                      n198 = case shown="真" w714 {
                        frame False {
                        }
                        frame True {
                          w719 = FALSE ("Δw1>C")
                          n199 = local write "Δw1>C"(w719) -> ()
                          n200 = local write "Δw2>C"(w719) -> ()
                          n201 = local write "θi"(0.0 ("θ")) -> ()
                        }
                      }
                    }
                  }
                }
              }
            }
            frame #11 {
              n202 = local write "正在测量"(FALSE) -> ()
            }
          }
          n203 = Build Array(w452, w451, w450, w449, w445) -> (w443:dbl[])
          n204 = local read "结果展示"() -> (w442:dbl[][])
          n205 = Insert Into Array(array=w442, new element=w443) -> (→"结果展示":dbl[][])  [unwired: 2 in]
        }
        n206 = Path To String(path=w122) -> (string=w129:string)
        n207 = Concatenate Strings(w129, "循环汇总" ("字符串"), ".xls" ("字符串")) -> (w109:string)
        n208 = String To Path(string=w109) -> (path=w128:path)
        n209 = call-poly <vilib>:"Write Delimited Spreadsheet.vi"("file path (dialog if empty)"=w128, "format (%.3f)"="%.16f", "2D data"=w120, "append to file? (new file:F)"=TRUE ("append to file? (F)"), "transpose? (no:F)"=FALSE ("transpose? (F)")) -> ()  [unwired: 9 in, 2 out]
        n210 = stacked-sequence {
          tunnel: w120 -> [_]
          tunnel: w119 -> [w158]
          tunnel: w118 -> [w157]
          tunnel: [w156] -> w117
          tunnel: [w155] -> w116
          tunnel: w113 -> [w154]
          tunnel: w112 -> [w153]
          tunnel: [w152] -> w111
          tunnel: [w151] -> w110
          tunnel: w109 -> [w150]
          tunnel: [w146] -> w100
          tunnel: [w145] -> w99
          frame #0 {
            n211 = stacked-sequence {
              seq-local: [_ _ w182 _ _] -> [_ _ _ w183 w197]
              seq-local: [w159 _ _ _ _] -> [_ _ _ _ w191]
              tunnel: [_ _ _ _ w193] -> _
              tunnel: w150 -> [w161 _ _ _ _]
              tunnel: [w159 _ _ _ _] -> w149
              tunnel: [_ _ _ _ w192] -> w148
              tunnel: [_ _ _ _ w191] -> w147
              frame #0 {
                n212 = Open Python Session(python version="3.9" ("Python version")) -> (session out=w168:refnum<k35>, error out=w166:errorcluster)  [unwired: 2 in]
                n213 = node(w168, path "D:/desktop/train/calloop.py" ("module path"), "Num_prediction" ("function name"), w166, 0.0, w161) -> (w167:refnum<k35>, w165:errorcluster, w159:dbl)  [unwired: 1 in, 2 out]
                "target angle" <- w159
                n214 = Close Python Session(session in=w167, error in=w165) -> ()  [unwired: 1 out]
              }
              frame #1 {
                n215 = Get Date/Time In Seconds() -> (seconds since 1Jan1904=w178:timestamp)
                n216 = Get Date/Time String(date format (0)=enum16{"short", "long", "abbreviated"}."abbreviated" ("日期格式(0)"), seconds (now)=w178, want seconds? (F)=TRUE ("需要秒？(F)")) -> (date string=w181:string, time string=w179:string)
                n217 = Search and Replace String(replace all?=TRUE ("替换全部？(F)"), input string=w179, search string=":" ("搜索字符串"), replace string="-" ("替换字符串(\"\")")) -> (result string=w180:string)  [unwired: 4 in, 3 out]
                n218 = Concatenate Strings("D:\\desktop\\train\\photo\\", w181, w180, "光谱" ("字符串"), ".jpg" ("字符串")) -> (→"图片地址 2":string)
              }
              frame #2 {
                # "SaveImage"
                n219 = local read "图片地址 2"() -> (w182:string)
              }
              frame #3 {
                n220 = Open Python Session(python version="3.9" ("Python version")) -> (session out=w190:refnum<k35>, error out=w188:errorcluster)  [unwired: 2 in]
                n221 = node(w190, path "D:/desktop/train/model/main.py" ("module path"), "screenshot" ("function name"), w188, w183) -> (w189:refnum<k35>, w187:errorcluster)  [unwired: 3 in, 2 out]
                n222 = Close Python Session(session in=w189, error in=w187) -> ()  [unwired: 1 out]
              }
              frame #4 {
                n223 = Open Python Session(python version="3.9" ("Python version")) -> (session out=w204:refnum<k35>, error out=w202:errorcluster)  [unwired: 2 in]
                n224 = node(w204, path "D:/desktop/train/newpro.py" ("module path"), "fun" ("function name"), w202, 0.0, w197) -> (w203:refnum<k35>, w201:errorcluster, w193:dbl)  [unwired: 1 in, 2 out]
                n225 = Close Python Session(session in=w203, error in=w201) -> ()  [unwired: 1 out]
                n226 = local write "current angle"(w193) -> ()
                n227 = Subtract(x=w193, y=w191) -> (x-y=w195:dbl)
                n228 = Absolute Value(x=w195) -> (abs(x)=w194:dbl)
                n229 = Less?(x=w194, y="误差值") -> (x < y?=w192:bool)
              }
            }
            n230 = while {
              shift-right: [w228] -> w156
              shift-left: w158 -> [w230]
              shift-right: [w227] -> w155
              shift-left: w157 -> [w229]
              shift-right: [w224] -> w152
              shift-left: w154 -> [w226]
              shift-right: [w223] -> w151
              shift-left: w153 -> [w225]
              tunnel: w149 -> [w222]
              tunnel: w148 -> [w221]
              shift-right: [w219] -> _
              shift-left: w147 -> [w220]
              tunnel: [w210] -> w146 mode=indexing
              tunnel: [w209] -> w145
              stop <- w206 stop-if-true
              n231 = stacked-sequence {
                seq-local: [_ w237 _ _ _ _ _ _] -> [_ _ w251 _ _ _ _ _]
                seq-local: [_ w236 _ _ _ _ _ _] -> [_ _ w250 _ _ _ _ _]
                seq-local: [_ _ _ _ w322 _ _ _] -> [_ _ _ _ _ _ w430 _]
                seq-local: [_ _ _ _ w321 _ _ _] -> [_ _ _ _ _ _ w429 _]
                seq-local: [_ w235 _ _ _ _ _ _] -> [_ _ _ _ _ w338 _ _]
                seq-local: [_ _ _ w262 _ _ _ _] -> [_ _ _ _ _ _ _ w436]
                tunnel: w230 -> [_ w239 _ _ _ _ _ _]
                tunnel: w229 -> [_ w238 _ _ _ _ _ _]
                tunnel: [_ _ w249 _ _ _ _ _] -> w228
                tunnel: [_ _ w248 _ _ _ _ _] -> w227
                tunnel: w226 -> [_ _ _ _ w324 _ _ _]
                tunnel: w225 -> [_ _ _ _ w323 _ _ _]
                tunnel: [_ _ _ _ _ _ w428 _] -> w224
                tunnel: [_ _ _ _ _ _ w427 _] -> w223
                tunnel: w222 -> [_ _ _ w263 _ _ _ _]
                tunnel: w220 -> [w231 _ _ _ _ _ _ _]
                tunnel: [_ _ _ w261 _ _ _ _] -> w219
                tunnel: [_ _ _ _ _ _ _ w436] -> w218
                tunnel: [_ _ _ w260 _ _ _ _] -> w217
                tunnel: [_ _ _ _ _ w337 _ _] -> w216
                tunnel: [_ _ _ _ _ w336 _ _] -> w215
                tunnel: [_ w235 _ _ _ _ _ _] -> w213
                tunnel: [_ _ _ _ _ w331 _ _] -> w214
                tunnel: [_ _ _ _ _ w330 _ _] -> w209
                frame #0 {
                  n232 = Less?(x=w231, y=10.0) -> (x < y?=w232:bool)
                  n233 = case shown="真" w232 {
                    frame False {
                    }
                    frame True {
                      n234 = local write "开光时间/ms"(u32 50 ("开光时间/ms")) -> ()
                    }
                  }
                }
                frame #1 {
                  n235 = flat-sequence {
                    tunnel: w239 -> [w247]
                    tunnel: w238 -> [w246]
                    tunnel: [w241] -> w237
                    tunnel: [w240] -> w236
                    frame #0 {
                      n236 = local read "channel输出口"() -> (w243:i32)
                      n237 = local write "Output"(TRUE ("布尔")) -> ()
                      n238 = Pick Line(multi-line string=":OUTP1 ON\n:OUTP2 ON" ("write buffer"), line index=w243) -> (output string=w242:string)  [unwired: 1 in]
                      n239 = VISA Write(VISA resource name=w247, write buffer=w242, error in (no error)=w246) -> (VISA resource name out=w241:refnum<visa-resource-name>, error out=w240:errorcluster)  [unwired: 1 out]
                    }
                  }
                  n240 = local read "开光时间/ms"() -> (w235:u32)
                  n241 = Wait (ms)(milliseconds to wait=w235) -> ()  [unwired: 1 out]
                }
                frame #2 {
                  n242 = flat-sequence {
                    tunnel: w251 -> [w259]
                    tunnel: w250 -> [w258]
                    tunnel: [w253] -> w249
                    tunnel: [w252] -> w248
                    frame #0 {
                      n243 = local read "channel输出口"() -> (w255:i32)
                      n244 = local write "Output"(TRUE ("布尔")) -> ()
                      n245 = Pick Line(multi-line string=":OUTP1 OFF\n:OUTP2 OFF" ("write buffer"), line index=w255) -> (output string=w254:string)  [unwired: 1 in]
                      n246 = VISA Write(VISA resource name=w259, write buffer=w254, error in (no error)=w258) -> (VISA resource name out=w253:refnum<visa-resource-name>, error out=w252:errorcluster)  [unwired: 1 out]
                    }
                  }
                }
                frame #3 {
                  n247 = stacked-sequence {
                    seq-local: [_ w280 _ _ _] -> [_ _ w281 w300 _]
                    seq-local: [_ _ _ w289 _] -> [_ _ _ _ w316]
                    tunnel: [_ _ _ _ w315] -> w264
                    tunnel: [_ _ _ w289 _] -> w260
                    frame #0 {
                      n248 = Get Date/Time In Seconds() -> (seconds since 1Jan1904=w276:timestamp)
                      n249 = Get Date/Time String(date format (0)=enum16{"short", "long", "abbreviated"}."abbreviated" ("日期格式(0)"), seconds (now)=w276, want seconds? (F)=TRUE ("需要秒？(F)")) -> (date string=w279:string, time string=w277:string)
                      n250 = Search and Replace String(replace all?=TRUE ("替换全部？(F)"), input string=w277, search string=":" ("搜索字符串"), replace string="-" ("替换字符串(\"\")")) -> (result string=w278:string)  [unwired: 4 in, 3 out]
                      n251 = Concatenate Strings("D:\\desktop\\train\\photo\\", w279, w278, "光谱" ("字符串"), ".jpg" ("字符串")) -> (→"图片地址 3":string)
                    }
                    frame #1 {
                      # "SaveImage"
                      n252 = local read "图片地址 3"() -> (w280:string)
                    }
                    frame #2 {
                      n253 = Open Python Session(python version="3.9" ("Python version")) -> (session out=w288:refnum<k35>, error out=w286:errorcluster)  [unwired: 2 in]
                      n254 = node(w288, path "D:/desktop/train/model/main.py" ("module path"), "screenshot" ("function name"), w286, w281) -> (w287:refnum<k35>, w285:errorcluster)  [unwired: 3 in, 2 out]
                      n255 = Close Python Session(session in=w287, error in=w285) -> ()  [unwired: 1 out]
                    }
                    frame #3 {
                      (unwired) 0 ("索引 (行)")
                      n256 = local read "结果展示"() -> (w294:dbl[][])
                      n257 = Open Python Session(python version="3.9" ("Python version")) -> (session out=w307:refnum<k35>, error out=w305:errorcluster)  [unwired: 2 in]
                      n258 = Array Size(array=w294) -> (size(s)=w299:i32[])
                      n259 = Index Array(array=w299, index=0 ("索引")) -> (element=w295:i32)
                      n260 = Decrement(x=w295) -> (x-1=w296:i32)
                      n261 = Index Array(array=w294, index (row)=w296, index (col)=0 ("禁用的索引 (列)")) -> (element=w293:dbl)
                      n262 = node(w307, path "D:/desktop/train/newpro.py" ("module path"), "fun" ("function name"), w305, 0.0, w300) -> (w306:refnum<k35>, w304:errorcluster, w289:dbl)  [unwired: 1 in, 2 out]
                      n263 = Subtract(x=w293, y=w289) -> (x-y=w292:dbl)
                      n264 = Greater?(x=w292, y=90.0) -> (0:w290:bool)
                      n265 = Close Python Session(session in=w306, error in=w304) -> ()  [unwired: 1 out]
                      n266 = case shown="真" w290 {
                        frame False {
                        }
                        frame True {
                          n267 = local read "数值"() -> (w310:i32)
                          n268 = Increment(x=w310) -> (x+1=→"数值":i32)
                        }
                      }
                    }
                    frame #4 {
                      n269 = local read "数值"() -> (w313:i32)
                      n270 = Quotient & Remainder(x=w313, y=2.0) -> (x-y*floor(x/y)=w312:dbl)  [unwired: 1 out]
                      n271 = Equal To 0?(x=w312) -> (x = 0?=w311:bool)
                      n272 = case shown="假" w311 {
                        tunnel: w316 -> [w319 w320]
                        tunnel: [w318 w320] -> w315
                        frame False {
                          n273 = Add(x=w319, y=180.0) -> (x+y=w318:dbl)
                        }
                        frame True {
                        }
                      }
                      n274 = local write "current angle"(w315) -> ()
                    }
                  }
                  n275 = local read "误差值"() -> (w265:dbl)
                  n276 = Subtract(x=w264, y=w263) -> (x-y=w261:dbl)
                  n277 = Absolute Value(x=w261) -> (abs(x)=w266:dbl)
                  n278 = Less?(x=w266, y=w265) -> (x < y?=w262:bool)
                }
                frame #4 {
                  w327 = " \u0001\u0001¢"  # Channel
                  n279 = Wait (ms)(milliseconds to wait=500) -> ()  [unwired: 1 out]
                  n280 = local write "照明光"(FALSE ("照明光")) -> ()
                  n281 = Concatenate Strings(w327, "\r") -> (w328:string)
                  n282 = VISA Write(VISA resource name=w324, write buffer=w328, error in (no error)=w323) -> (VISA resource name out=w322:refnum<visa-resource-name>, error out=w321:errorcluster)  [unwired: 1 out]
                }
                frame #5 {
                  n283 = local read "Area Number to Display"() -> (w384:i32)
                  n284 = local read "JYCCDLib.IJYCCDReqd"() -> (w380:refnum<k7>)
                  n285 = Get Date/Time In Seconds() -> (seconds since 1Jan1904=w332:timestamp)
                  n286 = local read "最终存储路径"() -> (w330:path)
                  n287 = Get Date/Time String(date format (0)=enum16{"short", "long", "abbreviated"}."abbreviated" ("日期格式(0)"), seconds (now)=w332, want seconds? (F)=TRUE ("需要秒？(F)")) -> (date string=w399:string, time string=w394:string)
                  n288 = call "MultiAccu - Acquire spectral.vi"("error in"=errorcluster {"status"=FALSE, "code"=0, "source"=""}, "Accumulations:"=u16 1, "ShutterOpen"=TRUE, "JYCCDLib.IJYCCDReqd"=w380) -> ("Acq Time(ms)"=w386:u32, "Array Out"=w385:i32[][][])  [unwired: 1 out]
                  n289 = local write "Acq Time(ms)"(w386) -> ()
                  n290 = local read "cut backlight"() -> (w369:bool)
                  n291 = local read "backlight"() -> (w367:bool)
                  n292 = Search and Replace String(replace all?=TRUE ("替换全部？(F)"), input string=w394, search string=":" ("搜索字符串"), replace string="-" ("替换字符串(\"\")")) -> (result string=w398:string)  [unwired: 4 in, 3 out]
                  n293 = Path To String(path=w330) -> (string=w389:string)
                  n294 = And(x=w369, y=w367) -> (x .and. y?=w368:bool)
                  n295 = call "Array reset dimension.vi"("Area Number"=w384, "Array In"=w385) -> ("Array Out"=w371:i32[][])
                  n296 = Concatenate Strings(w389, w399, w398, "光谱" ("字符串"), ".xls" ("字符串")) -> (w335:string)
                  n297 = case shown="假" w368 {
                    tunnel: [w423 w425] -> w370
                    tunnel: w371 -> [w423 w424]
                    frame False {
                    }
                    frame True {
                      n298 = local read "Backlight"() -> (w426:i32[][])
                      n299 = Subtract(x=w424, y=w426) -> (x-y=w425:i32[][])
                    }
                  }
                  n300 = String To Path(string=w335) -> (path=w403:path)
                  n301 = Format Date/Time String(time format string (%c)="%H%M%S" ("时间格式字符串(%c)"), seconds (now)=w332) -> (date/time string=w334:string)  [unwired: 1 in]
                  n302 = local write "Data"(w371) -> ()
                  n303 = local read "波长范围"() -> (w355:dbl[])
                  n304 = Index Array(array=w370, index (row)=0 ("索引 (行)")) -> (element=w404:i32[])  [unwired: 1 in]
                  n305 = Decimal String To Number(string=w334) -> (number=w331:i32)  [unwired: 2 in, 1 out]
                  n306 = local read "current angle"() -> (w354:dbl)
                  n307 = Reverse 1D Array(array=w404) -> (reversed array=w352:i32[])
                  n308 = local read "拟合起点"() -> (w362:i32)
                  n309 = local read "拟合终点"() -> (w364:i32)
                  n310 = call <vilib>:"Median Filter.vi"("left rank"=6, "X"=w352) -> ("Filtered X"=w348:dbl[])  [unwired: 8 in, 1 out]
                  n311 = Build Array(w354, w338, 0.0 ("元素")) -> (w353:dbl[])
                  n312 = Subtract(x=w364, y=w362) -> (x-y=w361:i32)
                  n313 = call "Convert to Dynamic Data3"("Array"=w355) -> ("Dynamic Data Type"=w377:dynamicdata)  [unwired: 3 in]
                  n314 = call "Convert to Dynamic Data4"("Array"=w352) -> ("Dynamic Data Type"=w376:dynamicdata)  [unwired: 3 in]
                  n315 = local read "滤波阈值"() -> (w339:dbl)
                  n316 = Array Subset(array=w355, index=w362, length=w361) -> (w360:dbl[])
                  n317 = call "Build XY Graph3"("Y Input"=w376, "X Input"=w377) -> ("XY Graph"=w349:cluster{"Y":dbl[], "Y":dbl[]}[])  [unwired: 8 in, 1 out]
                  n318 = call "转换至动态数据6"("Array"=w360) -> ("Dynamic Data Type"=w374:dynamicdata)  [unwired: 3 in]
                  n319 = local write "Spectrum"(w349) -> ()
                  n320 = In Range and Coerce(upper limit=w339, x=w348, lower limit=-100.0) -> (In Range?=w343:bool[])  [unwired: 1 out]
                  n321 = local write "范围内？"(w343) -> ()
                  n322 = Not(x=w343) -> (.not. x?=w365:bool[])
                  n323 = Or Array Elements(Boolean array=w365) -> (logical OR=w346:bool)
                  n324 = local read "X Pixels:"() -> (w347:i32)
                  n325 = local read "波长范围"() -> (w356:dbl[])
                  n326 = local read "滤波阈值"() -> (w345:dbl)
                  n327 = case shown="真" w346 {
                    tunnel: w348 -> [w406 w410]
                    tunnel: w347 -> [_ w409]
                    tunnel: w345 -> [_ w408]
                    tunnel: [w406 w407] -> w344
                    frame False {
                    }
                    frame True {
                      n328 = for {
                        N: w409 -> [_]
                        tunnel: w410 -> [w414] mode=indexing
                        tunnel: [w413] -> w407 mode=indexing
                        shift-right: [w413] -> _
                        shift-left: _ -> [w412]
                        tunnel: w408 -> [w411]
                        n329 = Greater?(x=w414, y=w411) -> (0:w416:bool)
                        n330 = Less?(x=w414, y=-100.0) -> (x < y?=w417:bool)
                        n331 = Or(x=w416, y=w417) -> (x .or. y?=w415:bool)
                        n332 = case shown="真" w415 {
                          tunnel: w414 -> [w419 _]
                          tunnel: [w419 w421] -> w413
                          tunnel: w412 -> [_ w422]
                          frame False {
                          }
                          frame True {
                            n333 = call <vilib>:"Median Filter PtByPt.vi"("rank"=5, "x"=w422) -> ("Filtered x"=w421:dbl)  [unwired: 2 in, 1 out]
                          }
                        }
                      }
                    }
                  }
                  n334 = Array Subset(array=w344, index=w362, length=w361) -> (w363:dbl[])
                  n335 = call "转换至动态数据5"("Array"=w363) -> ("Dynamic Data Type"=w375:dynamicdata)  [unwired: 3 in]
                  n336 = call "曲线拟合3"("Locations"=w374, "Signals"=w375) -> ("best fit"=w379:dynamicdata, "non-linear coefficients"=w378:dynamicdata)  [unwired: 5 in, 3 out]
                  n337 = call "从动态数据转换5"("Dynamic Data Type"=w378) -> ("Array"=w342:dbl[])  [unwired: 3 in]
                  n338 = call "从动态数据转换6"("Dynamic Data Type"=w379) -> ("Array"=w350:dbl[])  [unwired: 3 in]
                  n339 = Build Array(w355, w348, w350, w342, w353) -> (w405:dbl[][])
                  n340 = call-poly <vilib>:"Write Delimited Spreadsheet.vi"("file path (dialog if empty)"=w403, "format (%.3f)"="%.16f", "2D data"=w405, "append to file? (new file:F)"=TRUE ("append to file? (F)"), "transpose? (no:F)"=TRUE ("transpose? (F)")) -> ()  [unwired: 9 in, 2 out]
                  n341 = Index Array(array=w342, index #1=0 ("索引"), index #2=1 ("索引")) -> (element #1=w341:dbl, element #2=w340:dbl)
                  n342 = local write "拟合参数"(w342) -> ()
                  n343 = Bundle("波长范围"=w356, "Filtered X"=w344) -> (w359:cluster{"波长范围 ":dbl[], "Filtered X":dbl[]})  [unwired: 1 in]
                  n344 = Bundle(w360, "Array"=w350) -> (w358:cluster{dbl[], "Array":dbl[]})  [unwired: 1 in]
                  n345 = Array Max & Min(array=w350) -> (max value=w336:dbl)  [unwired: 3 out]
                  n346 = Array Max & Min(array=w344) -> (max value=w337:dbl)  [unwired: 3 out]
                  n347 = local write "xc"(w341) -> ()
                  n348 = local write "w"(w340) -> ()
                  n349 = Build Array(w359, w358) -> (w357:cluster{"波长范围 ":dbl[], "Array":dbl[]}[])
                  n350 = local write "拟合峰值"(w336) -> ()
                  n351 = local write "原始峰值"(w337) -> ()
                  n352 = local write "best fit"(w357) -> ()
                }
                frame #6 {
                  w433 = " \u0001\u0000¡"  # Channel
                  n353 = Concatenate Strings(w433, "\r") -> (w434:string)
                  n354 = local write "照明光"(TRUE ("照明光")) -> ()
                  n355 = VISA Write(VISA resource name=w430, write buffer=w434, error in (no error)=w429) -> (VISA resource name out=w428:refnum<visa-resource-name>, error out=w427:errorcluster)  [unwired: 1 out]
                  n356 = Wait (ms)(milliseconds to wait=1200) -> ()  [unwired: 1 out]
                }
                frame #7 {
                }
              }
              n357 = Or(x=w221, y=w218) -> (x .or. y?=w207:bool)
              n358 = local read "结果展示"() -> (w211:dbl[][])
              n359 = Build Array(w217, w216, w215, w214, w213) -> (w210:dbl[])
              n360 = Insert Into Array(array=w211, new element=w210) -> (w212:dbl[][])  [unwired: 2 in]
              n361 = Or(x="停止预测", y=w207) -> (x .or. y?=w206:bool)
              n362 = local write "结果展示"(w212) -> ()
            }
          }
        }
        n363 = local write "结果展示"(dbl[][] [] ("结果展示")) -> ()
        n364 = Path To String(path=w99) -> (string=w108:string)
        n365 = local write "停止预测"(FALSE ("停止预测")) -> ()
        n366 = local write "数值"(0 ("数值")) -> ()
        n367 = VISA Close(VISA resource name=w111, error in (no error)=w110) -> (error out=→"照明光error out":errorcluster)
        n368 = VISA Close(VISA resource name=w117, error in (no error)=w116) -> (error out=→"output control error":errorcluster)
        n369 = Concatenate Strings(w108, "验证汇总" ("字符串"), ".xls" ("字符串")) -> (w101:string)
        n370 = String To Path(string=w101) -> (path=w107:path)
        n371 = call-poly <vilib>:"Write Delimited Spreadsheet.vi"("file path (dialog if empty)"=w107, "format (%.3f)"="%.16f", "2D data"=w100, "append to file? (new file:F)"=TRUE ("append to file? (F)"), "transpose? (no:F)"=FALSE ("transpose? (F)")) -> ()  [unwired: 9 in, 2 out]
      }
    }
    n372 = event shown="[1] \"低电平持续输出\": 值改变" {
      selector: _ -> [_ _]
      dyn-events: _ -> [_ _]
      timeout: u32 0 ("Time") -> [_ _]
      tunnel: "低电平持续输出" -> [_ w793]
      event Timeout {
        n373 = event-data() -> ()  [unwired: 1 in, 2 out]
      }
      event "低电平持续输出": Value Change {
        w797 = " :SOUR1\n :SOUR2"  # Channel
        n374 = event-data() -> ()  [unwired: 1 in, 6 out]
        n375 = local read "channel输出口"() -> (w798:i32)
        n376 = Pick Line(multi-line string=w797, line index=w798) -> (output string=w796:string)  [unwired: 1 in]
        n377 = local read "VISA 信号发生器"() -> (w801:refnum<visa-resource-name>)
        n378 = VISA Open(VISA resource name=w801) -> (VISA resource name=w800:refnum<visa-resource-name>, error out=w799:errorcluster)  [unwired: 4 in]
        n379 = stacked-sequence {
          seq-local: [w807 _ _ _ _ _ _ _ _ _ _ _ _] -> [_ _ w822 _ _ _ _ _ _ _ _ _ _]
          seq-local: [w806 _ _ _ _ _ _ _ _ _ _ _ _] -> [_ _ w821 _ _ _ _ _ _ _ _ _ _]
          seq-local: [_ _ w820 _ _ _ _ _ _ _ _ _ _] -> [_ _ _ _ w825 _ _ _ _ _ _ _ _]
          seq-local: [_ _ w819 _ _ _ _ _ _ _ _ _ _] -> [_ _ _ _ w826 _ _ _ _ _ _ _ _]
          seq-local: [_ _ _ _ w834 _ _ _ _ _ _ _ _] -> [_ _ _ _ _ _ w845 _ _ _ _ _ _]
          seq-local: [_ _ _ _ w833 _ _ _ _ _ _ _ _] -> [_ _ _ _ _ _ w844 _ _ _ _ _ _]
          seq-local: [_ _ _ _ _ _ w838 _ _ _ _ _ _] -> [_ _ _ _ _ _ _ _ w848 _ _ _ _]
          seq-local: [_ _ _ _ _ _ w837 _ _ _ _ _ _] -> [_ _ _ _ _ _ _ _ w847 _ _ _ _]
          seq-local: [_ _ _ _ _ _ _ _ w851 _ _ _ _] -> [_ _ _ _ _ _ _ _ _ _ w862 _ _]
          seq-local: [_ _ _ _ _ _ _ _ w850 _ _ _ _] -> [_ _ _ _ _ _ _ _ _ _ w861 _ _]
          seq-local: [_ _ _ _ _ _ _ _ _ _ w859 _ _] -> [_ _ _ _ _ _ _ _ _ _ _ _ w876]
          seq-local: [_ _ _ _ _ _ _ _ _ _ w858 _ _] -> [_ _ _ _ _ _ _ _ _ _ _ _ w875]
          tunnel: w800 -> [w812 _ _ _ _ _ _ _ _ _ _ _ _]
          tunnel: w799 -> [w805 _ _ _ _ _ _ _ _ _ _ _ _]
          tunnel: w796 -> [w804 _ w818 _ w831 _ w842 _ w852 _ w865 _ _]
          tunnel: [_ _ _ _ _ _ _ _ _ _ _ _ w874] -> w795
          tunnel: [_ _ _ _ _ _ _ _ _ _ _ _ w872] -> w794
          tunnel: w793 -> [_ _ _ _ _ _ _ _ _ _ _ _ w873]
          frame #0 {
            w809 = " PULSe"  # Function Command
            n380 = local read "输出信号波形"() -> (w803:u16)
            n381 = Concatenate Strings(w804, ":FUNC" ("string (\"\")")) -> (w810:string)
            n382 = Pick Line(string ("")=w810, multi-line string=w809, line index=w803) -> (output string=w808:string)
            n383 = VISA Write(VISA resource name=w812, write buffer=w808, error in (no error)=w805) -> (VISA resource name out=w807:refnum<visa-resource-name>, error out=w806:errorcluster)  [unwired: 1 out]
          }
          frame #1 {
            n384 = Wait (ms)(milliseconds to wait=u32 150) -> ()  [unwired: 1 out]
          }
          frame #2 {
            n385 = Number To Fractional String(use system decimal point (T)=TRUE ("使用系统小数点(T)"), number=1.0 ("数字")) -> (F-format string=w816:string)  [unwired: 2 in]
            n386 = Concatenate Strings ("连接字符串")(w818, ":VOLTage：HIGH ", w816) -> (w815:string)
            n387 = VISA Write(VISA resource name=w822, write buffer=w815, error in (no error)=w821) -> (VISA resource name out=w820:refnum<visa-resource-name>, error out=w819:errorcluster)  [unwired: 1 out]
          }
          frame #3 {
            n388 = Wait (ms)(milliseconds to wait=u32 150) -> ()  [unwired: 1 out]
          }
          frame #4 {
            # "1 电压偏置"
            n389 = Number To Fractional String(use system decimal point (T)=TRUE ("使用系统小数点(T)"), number=0.0 ("数字")) -> (F-format string=w829:string)  [unwired: 2 in]
            n390 = Concatenate Strings(w831, ":VOLTage:LOW ", w829) -> (w830:string)
            n391 = VISA Write(VISA resource name=w825, write buffer=w830, error in (no error)=w826) -> (VISA resource name out=w834:refnum<visa-resource-name>, error out=w833:errorcluster)  [unwired: 1 out]
          }
          frame #5 {
            n392 = Wait (ms)(milliseconds to wait=u32 150) -> ()  [unwired: 1 out]
          }
          frame #6 {
            n393 = local read "channel输出口"() -> (w840:i32)
            n394 = Pick Line(multi-line string=":OUTP1:IMPedance \n:OUTP2:IMPedance " ("write buffer"), line index=w840) -> (output string=w839:string)  [unwired: 1 in]
            n395 = Concatenate Strings ("连接字符串")(w842, w839, "INFINITY") -> (w843:string)
            n396 = VISA Write(VISA resource name=w845, write buffer=w843, error in (no error)=w844) -> (VISA resource name out=w838:refnum<visa-resource-name>, error out=w837:errorcluster)  [unwired: 1 out]
          }
          frame #7 {
            n397 = Wait (ms)(milliseconds to wait=u32 150) -> ()  [unwired: 1 out]
          }
          frame #8 {
            n398 = Number To Fractional String(use system decimal point (T)=TRUE ("使用系统小数点(T)"), number=0.0 ("数字")) -> (F-format string=w855:string)  [unwired: 2 in]
            n399 = Concatenate Strings(w852, ":PULSe:DELay ", w855) -> (w853:string)
            n400 = VISA Write(VISA resource name=w848, write buffer=w853, error in (no error)=w847) -> (VISA resource name out=w851:refnum<visa-resource-name>, error out=w850:errorcluster)  [unwired: 1 out]
          }
          frame #9 {
            n401 = Wait (ms)(milliseconds to wait=u32 150) -> ()  [unwired: 1 out]
          }
          frame #10 {
            w866 = ":LEADing\n:TRAiling "  # Channel
            w870 = ":PULSe:TRANsition"  # VOLTage:Offset
            n402 = local read "上升下降沿"() -> (w867:i32)
            n403 = Pick Line(multi-line string=w866, line index=w867) -> (output string=w863:string)  [unwired: 1 in]
            n404 = Number To Fractional String(use system decimal point (T)=TRUE ("使用系统小数点(T)"), number=0.0 ("数字")) -> (F-format string=w864:string)  [unwired: 2 in]
            n405 = Concatenate Strings(w865, w870, w863, w864) -> (w868:string)
            n406 = VISA Write(VISA resource name=w862, write buffer=w868, error in (no error)=w861) -> (VISA resource name out=w859:refnum<visa-resource-name>, error out=w858:errorcluster)  [unwired: 1 out]
          }
          frame #11 {
            n407 = Wait (ms)(milliseconds to wait=u32 150) -> ()  [unwired: 1 out]
          }
          frame #12 {
            n408 = case shown="假" w873 {
              tunnel: w876 -> [w884 w885]
              tunnel: [w883 w892] -> w872
              tunnel: w875 -> [w882 w890]
              tunnel: [w881 w891] -> w874
              frame True {
                n409 = local write "Output"(TRUE ("布尔")) -> ()
                n410 = local read "channel输出口"() -> (w878:i32)
                n411 = Pick Line(multi-line string=":OUTP1 ON\n:OUTP2 ON" ("write buffer"), line index=w878) -> (output string=w877:string)  [unwired: 1 in]
                n412 = VISA Write(VISA resource name=w884, write buffer=w877, error in (no error)=w882) -> (VISA resource name out=w881:refnum<visa-resource-name>, error out=w883:errorcluster)  [unwired: 1 out]
              }
              frame False {
                n413 = local read "channel输出口"() -> (w887:i32)
                n414 = Pick Line(multi-line string=":OUTP1 OFF\n:OUTP2 OFF" ("write buffer"), line index=w887) -> (output string=w886:string)  [unwired: 1 in]
                n415 = VISA Write(VISA resource name=w885, write buffer=w886, error in (no error)=w890) -> (VISA resource name out=w891:refnum<visa-resource-name>, error out=w892:errorcluster)  [unwired: 1 out]
                n416 = local write "Output"(FALSE ("布尔")) -> ()
              }
            }
          }
        }
        n417 = VISA Close(VISA resource name=w795, error in (no error)=w794) -> (error out=→"output control error  4":errorcluster)
      }
    }
    n418 = event shown="[1] \"Enable\": 值改变" {
      selector: _ -> [_ _]
      dyn-events: _ -> [_ _]
      timeout: u32 0 ("Time") -> [_ _]
      tunnel: "Enable" -> [_ w768]
      event Timeout {
        n419 = event-data() -> ()  [unwired: 1 in, 2 out]
      }
      event "Enable": Value Change {
        n420 = event-data() -> ()  [unwired: 1 in, 6 out]
        n421 = local read "VISA 信号发生器"() -> (w764:refnum<visa-resource-name>)
        n422 = VISA Open(VISA resource name=w764) -> (VISA resource name=w767:refnum<visa-resource-name>, error out=w770:errorcluster)  [unwired: 4 in]
        n423 = stacked-sequence {
          tunnel: w768 -> [w775 _]
          tunnel: w770 -> [w774 _]
          tunnel: w767 -> [w773 _]
          tunnel: [w772 _] -> w766
          tunnel: [w771 _] -> w765
          frame #0 {
            n424 = case shown="真" w775 {
              tunnel: w773 -> [w783 w791]
              tunnel: [w782 w790] -> w771
              tunnel: w774 -> [w781 w788]
              tunnel: [w780 w789] -> w772
              frame True {
                n425 = local write "Output"(TRUE ("布尔")) -> ()
                n426 = local read "channel输出口"() -> (w777:i32)
                n427 = Pick Line(multi-line string=":OUTP1 ON\n:OUTP2 ON" ("write buffer"), line index=w777) -> (output string=w776:string)  [unwired: 1 in]
                n428 = VISA Write(VISA resource name=w783, write buffer=w776, error in (no error)=w781) -> (VISA resource name out=w780:refnum<visa-resource-name>, error out=w782:errorcluster)  [unwired: 1 out]
              }
              frame False {
                n429 = local read "channel输出口"() -> (w785:i32)
                n430 = Pick Line(multi-line string=":OUTP1 OFF\n:OUTP2 OFF" ("write buffer"), line index=w785) -> (output string=w784:string)  [unwired: 1 in]
                n431 = VISA Write(VISA resource name=w791, write buffer=w784, error in (no error)=w788) -> (VISA resource name out=w789:refnum<visa-resource-name>, error out=w790:errorcluster)  [unwired: 1 out]
                n432 = local write "Output"(FALSE ("布尔")) -> ()
              }
            }
          }
          frame #1 {
            n433 = Wait (ms)(milliseconds to wait=u32 150) -> ()  [unwired: 1 out]
          }
        }
        n434 = VISA Close(VISA resource name=w766, error in (no error)=w765) -> (error out=→"output control error  5":errorcluster)
      }
    }
    n435 = event shown="[1] \"Enable 2\": 值改变" {
      selector: _ -> [_ _]
      dyn-events: _ -> [_ _]
      timeout: u32 0 ("Time") -> [_ _]
      tunnel: "Enable 2" -> [_ w28]
      event Timeout {
        n436 = event-data() -> ()  [unwired: 1 in, 2 out]
      }
      event "Enable 2": Value Change {
        n437 = event-data() -> ()  [unwired: 1 in, 6 out]
        n438 = Not(x=w28) -> (.not. x?=w27:bool)
        n439 = local read "VISA 信号发生器"() -> (w29:refnum<visa-resource-name>)
        n440 = VISA Open(VISA resource name=w29) -> (VISA resource name=w32:refnum<visa-resource-name>, error out=w33:errorcluster)  [unwired: 4 in]
        n441 = stacked-sequence {
          tunnel: w27 -> [w38 _]
          tunnel: w33 -> [w37 _]
          tunnel: w32 -> [w36 _]
          tunnel: [w35 _] -> w31
          tunnel: [w34 _] -> w30
          frame #0 {
            n442 = case shown="真" w38 {
              tunnel: w36 -> [w47 w58]
              tunnel: [w46 w57] -> w34
              tunnel: w37 -> [w45 w55]
              tunnel: [w44 w56] -> w35
              frame True {
                n443 = local read "channel输出口"() -> (w40:i32)
                n444 = local write "Output 2"(FALSE ("布尔")) -> ()
                n445 = case shown="1" w40 {
                  tunnel: [1 0] -> w39
                  frame 0, Default {
                  }
                  frame 1 {
                  }
                }
                n446 = Pick Line(multi-line string=":OUTP1 ON\n:OUTP2 ON" ("write buffer"), line index=w39) -> (output string=w41:string)  [unwired: 1 in]
                n447 = VISA Write(VISA resource name=w47, write buffer=w41, error in (no error)=w45) -> (VISA resource name out=w44:refnum<visa-resource-name>, error out=w46:errorcluster)  [unwired: 1 out]
              }
              frame False {
                n448 = local read "channel输出口"() -> (w51:i32)
                n449 = case shown="1" w51 {
                  tunnel: [1 0] -> w50
                  frame 0, Default {
                  }
                  frame 1 {
                  }
                }
                n450 = Pick Line(multi-line string=":OUTP1 OFF\n:OUTP2 OFF" ("write buffer"), line index=w50) -> (output string=w52:string)  [unwired: 1 in]
                n451 = VISA Write(VISA resource name=w58, write buffer=w52, error in (no error)=w55) -> (VISA resource name out=w56:refnum<visa-resource-name>, error out=w57:errorcluster)  [unwired: 1 out]
                n452 = local write "Output 2"(TRUE ("布尔")) -> ()
              }
            }
          }
          frame #1 {
            n453 = Wait (ms)(milliseconds to wait=u32 150) -> ()  [unwired: 1 out]
          }
        }
        n454 = VISA Close(VISA resource name=w31, error in (no error)=w30) -> ()  [unwired: 1 out]
      }
    }
    n455 = case shown="真" "设置参数" {
      frame False {
      }
      frame True {
        w899 = " :SOUR1\n :SOUR2"  # Channel
        n456 = local read "VISA 信号发生器"() -> (w901:refnum<visa-resource-name>)
        n457 = local read "channel输出口"() -> (w900:i32)
        n458 = case shown="1" w900 {
          tunnel: [1 0] -> w893
          frame 0, Default {
          }
          frame 1 {
          }
        }
        n459 = VISA Open(VISA resource name=w901) -> (VISA resource name=w904:refnum<visa-resource-name>, error out=w905:errorcluster)  [unwired: 4 in]
        n460 = Pick Line(multi-line string=w899, line index=w893) -> (output string=w894:string)  [unwired: 1 in]
        n461 = Pick Line(multi-line string=w899, line index=w900) -> (output string=w902:string)  [unwired: 1 in]
        n462 = stacked-sequence {
          seq-local: [w1001 _ _ _ _ _ _ _ _ _ _ _ _ _ _] -> [_ _ w1016 _ _ _ _ _ _ _ _ _ _ _ _]
          seq-local: [w1000 _ _ _ _ _ _ _ _ _ _ _ _ _ _] -> [_ _ w1015 _ _ _ _ _ _ _ w1054 _ _ _ _]
          seq-local: [_ _ w1014 _ _ _ _ _ _ _ _ _ _ _ _] -> [_ _ _ _ w1025 _ _ _ _ _ _ _ _ _ _]
          seq-local: [_ _ w1013 _ _ _ _ _ _ _ _ _ _ _ _] -> [_ _ _ _ w1024 _ _ _ _ _ _ _ _ _ _]
          seq-local: [_ _ _ _ w1023 _ _ _ _ _ _ _ _ _ _] -> [_ _ _ _ _ _ w1031 _ _ _ _ _ _ _ _]
          seq-local: [_ _ _ _ w1020 _ _ _ _ _ _ _ _ _ _] -> [_ _ _ _ _ _ w1030 _ _ _ _ _ _ _ _]
          seq-local: [_ _ _ _ _ _ w1038 _ _ _ _ _ _ _ _] -> [_ _ _ _ _ _ _ _ w1049 _ _ _ _ _ _]
          seq-local: [_ _ _ _ _ _ w1037 _ _ _ _ _ _ _ _] -> [_ _ _ _ _ _ _ _ w1048 _ _ _ _ _ _]
          seq-local: [_ _ _ _ _ _ _ _ w1042 _ _ _ _ _ _] -> [_ _ _ _ _ _ _ _ _ _ w1055 _ _ _ _]
          seq-local: [_ _ _ _ _ _ _ _ w1041 _ _ _ _ _ _] -> [_ _ _ _ _ _ _ _ _ _ _ _ _ _ _]
          seq-local: [_ _ _ _ _ _ _ _ _ _ w1051 _ _ _ _] -> [_ _ _ _ _ _ _ _ _ _ _ _ w1065 _ _]
          seq-local: [_ _ _ _ _ _ _ _ _ _ w1052 _ _ _ _] -> [_ _ _ _ _ _ _ _ _ _ _ _ w1064 _ _]
          seq-local: [_ _ _ _ _ _ _ _ _ _ _ _ w1063 _ _] -> [_ _ _ _ _ _ _ _ _ _ _ _ _ _ w1076]
          seq-local: [_ _ _ _ _ _ _ _ _ _ _ _ w1062 _ _] -> [_ _ _ _ _ _ _ _ _ _ _ _ _ _ w1075]
          tunnel: w904 -> [w1006 _ _ _ _ _ _ _ _ _ _ _ _ _ _]
          tunnel: w905 -> [w999 _ _ _ _ _ _ _ _ _ _ _ _ _ _]
          tunnel: w902 -> [w998 _ w1012 _ w1019 _ w1035 _ w1046 _ w1056 _ w1066 _ w1079]
          tunnel: [_ _ _ _ _ _ _ _ _ _ _ _ _ _ w1074] -> w898
          tunnel: [_ _ _ _ _ _ _ _ _ _ _ _ _ _ w1073] -> w897
          frame #0 {
            w1003 = " PULSe"  # Function Command
            n463 = local read "输出信号波形"() -> (w997:u16)
            n464 = Concatenate Strings(w998, ":FUNC" ("string (\"\")")) -> (w1004:string)
            n465 = Pick Line(string ("")=w1004, multi-line string=w1003, line index=w997) -> (output string=w1002:string)
            n466 = VISA Write(VISA resource name=w1006, write buffer=w1002, error in (no error)=w999) -> (VISA resource name out=w1001:refnum<visa-resource-name>, error out=w1000:errorcluster)  [unwired: 1 out]
          }
          frame #1 {
            n467 = Wait (ms)(milliseconds to wait=u32 150) -> ()  [unwired: 1 out]
          }
          frame #2 {
            n468 = Number To Fractional String(use system decimal point (T)=TRUE ("使用系统小数点(T)"), number="低电平/V") -> (F-format string=w1010:string)  [unwired: 2 in]
            n469 = Concatenate Strings ("连接字符串")(w1012, ":VOLTage:LOW ", w1010) -> (w1009:string)
            n470 = VISA Write(VISA resource name=w1016, write buffer=w1009, error in (no error)=w1015) -> (VISA resource name out=w1014:refnum<visa-resource-name>, error out=w1013:errorcluster)  [unwired: 1 out]
          }
          frame #3 {
            n471 = Wait (ms)(milliseconds to wait=u32 150) -> ()  [unwired: 1 out]
          }
          frame #4 {
            # "1 频率"
            n472 = Concatenate Strings(w1019, ":FREQ ") -> (w1026:string)
            n473 = Format Into String ("格式化写入字符串")(initial string=w1026, "频率/Hz") -> (resulting string=w1027:string)  [unwired: 2 in, 1 out]
            n474 = VISA Write(VISA resource name=w1025, write buffer=w1027, error in (no error)=w1024) -> (VISA resource name out=w1023:refnum<visa-resource-name>, error out=w1020:errorcluster)  [unwired: 1 out]
          }
          frame #5 {
            n475 = Wait (ms)(milliseconds to wait=u32 150) -> ()  [unwired: 1 out]
          }
          frame #6 {
            n476 = Number To Fractional String(use system decimal point (T)=TRUE ("使用系统小数点(T)"), number="高电平/V") -> (F-format string=w1032:string)  [unwired: 2 in]
            n477 = Concatenate Strings(w1035, ":VOLTage:HIGH ", w1032) -> (w1034:string)
            n478 = VISA Write(VISA resource name=w1031, write buffer=w1034, error in (no error)=w1030) -> (VISA resource name out=w1038:refnum<visa-resource-name>, error out=w1037:errorcluster)  [unwired: 1 out]
          }
          frame #7 {
            n479 = Wait (ms)(milliseconds to wait=u32 150) -> ()  [unwired: 1 out]
          }
          frame #8 {
            n480 = local read "channel输出口"() -> (w1044:i32)
            n481 = Pick Line(multi-line string=":OUTP1:IMPedance \n:OUTP2:IMPedance " ("write buffer"), line index=w1044) -> (output string=w1043:string)  [unwired: 1 in]
            n482 = Concatenate Strings ("连接字符串")(w1046, w1043, "INFINITY") -> (w1047:string)
            n483 = VISA Write(VISA resource name=w1049, write buffer=w1047, error in (no error)=w1048) -> (VISA resource name out=w1042:refnum<visa-resource-name>, error out=w1041:errorcluster)  [unwired: 1 out]
          }
          frame #9 {
            n484 = Wait (ms)(milliseconds to wait=u32 150) -> ()  [unwired: 1 out]
          }
          frame #10 {
            n485 = Number To Fractional String(use system decimal point (T)=TRUE ("使用系统小数点(T)"), number="占空比/%") -> (F-format string=w1058:string)  [unwired: 2 in]
            n486 = Concatenate Strings(w1056, ":PULSe:DCYCle ", w1058) -> (w1053:string)
            n487 = VISA Write(VISA resource name=w1055, write buffer=w1053, error in (no error)=w1054) -> (VISA resource name out=w1051:refnum<visa-resource-name>, error out=w1052:errorcluster)  [unwired: 1 out]
          }
          frame #11 {
            n488 = Wait (ms)(milliseconds to wait=u32 150) -> ()  [unwired: 1 out]
          }
          frame #12 {
            n489 = Number To Fractional String(use system decimal point (T)=TRUE ("使用系统小数点(T)"), number="延时/s") -> (F-format string=w1069:string)  [unwired: 2 in]
            n490 = Concatenate Strings(w1066, ":PULSe:DELay ", w1069) -> (w1067:string)
            n491 = VISA Write(VISA resource name=w1065, write buffer=w1067, error in (no error)=w1064) -> (VISA resource name out=w1063:refnum<visa-resource-name>, error out=w1062:errorcluster)  [unwired: 1 out]
          }
          frame #13 {
            n492 = Wait (ms)(milliseconds to wait=u32 150) -> ()  [unwired: 1 out]
          }
          frame #14 {
            w1080 = ":LEADing\n:TRAiling "  # Channel
            w1085 = ":PULSe:TRANsition"  # VOLTage:Offset
            n493 = local read "上升下降沿"() -> (w1081:i32)
            n494 = Pick Line(multi-line string=w1080, line index=w1081) -> (output string=w1077:string)  [unwired: 1 in]
            n495 = Number To Fractional String(use system decimal point (T)=TRUE ("使用系统小数点(T)"), number="上升下降沿/s") -> (F-format string=w1078:string)  [unwired: 2 in]
            n496 = Concatenate Strings(w1079, w1085, w1077, w1078) -> (w1082:string)
            n497 = VISA Write(VISA resource name=w1076, write buffer=w1082, error in (no error)=w1075) -> (VISA resource name out=w1074:refnum<visa-resource-name>, error out=w1073:errorcluster)  [unwired: 1 out]
          }
        }
        n498 = stacked-sequence {
          seq-local: [w912 _ _ _ _ _ _ _ _ _ _ _ _ _ _] -> [_ _ w927 _ _ _ _ _ _ _ _ _ _ _ _]
          seq-local: [w911 _ _ _ _ _ _ _ _ _ _ _ _ _ _] -> [_ _ w926 _ _ _ _ _ _ _ w965 _ _ _ _]
          seq-local: [_ _ w925 _ _ _ _ _ _ _ _ _ _ _ _] -> [_ _ _ _ w936 _ _ _ _ _ _ _ _ _ _]
          seq-local: [_ _ w924 _ _ _ _ _ _ _ _ _ _ _ _] -> [_ _ _ _ w935 _ _ _ _ _ _ _ _ _ _]
          seq-local: [_ _ _ _ w934 _ _ _ _ _ _ _ _ _ _] -> [_ _ _ _ _ _ w942 _ _ _ _ _ _ _ _]
          seq-local: [_ _ _ _ w931 _ _ _ _ _ _ _ _ _ _] -> [_ _ _ _ _ _ w941 _ _ _ _ _ _ _ _]
          seq-local: [_ _ _ _ _ _ w949 _ _ _ _ _ _ _ _] -> [_ _ _ _ _ _ _ _ w960 _ _ _ _ _ _]
          seq-local: [_ _ _ _ _ _ w948 _ _ _ _ _ _ _ _] -> [_ _ _ _ _ _ _ _ w959 _ _ _ _ _ _]
          seq-local: [_ _ _ _ _ _ _ _ w954 _ _ _ _ _ _] -> [_ _ _ _ _ _ _ _ _ _ w966 _ _ _ _]
          seq-local: [_ _ _ _ _ _ _ _ w953 _ _ _ _ _ _] -> [_ _ _ _ _ _ _ _ _ _ _ _ _ _ _]
          seq-local: [_ _ _ _ _ _ _ _ _ _ w962 _ _ _ _] -> [_ _ _ _ _ _ _ _ _ _ _ _ w976 _ _]
          seq-local: [_ _ _ _ _ _ _ _ _ _ w963 _ _ _ _] -> [_ _ _ _ _ _ _ _ _ _ _ _ w975 _ _]
          seq-local: [_ _ _ _ _ _ _ _ _ _ _ _ w974 _ _] -> [_ _ _ _ _ _ _ _ _ _ _ _ _ _ w989]
          seq-local: [_ _ _ _ _ _ _ _ _ _ _ _ w973 _ _] -> [_ _ _ _ _ _ _ _ _ _ _ _ _ _ w988]
          tunnel: w898 -> [w917 _ _ _ _ _ _ _ _ _ _ _ _ _ _]
          tunnel: w897 -> [w910 _ _ _ _ _ _ _ _ _ _ _ _ _ _]
          tunnel: w894 -> [w909 _ w923 _ w930 _ w946 _ w957 _ w967 _ w977 _ w984]
          tunnel: [_ _ _ _ _ _ _ _ _ _ _ _ _ _ w987] -> w896
          tunnel: [_ _ _ _ _ _ _ _ _ _ _ _ _ _ w986] -> w895
          tunnel: w893 -> [_ _ _ _ _ _ _ _ w951 _ _ _ _ _ _]
          frame #0 {
            w914 = " PULSe"  # Function Command
            n499 = Concatenate Strings(w909, ":FUNC" ("string (\"\")")) -> (w915:string)
            n500 = Pick Line(string ("")=w915, multi-line string=w914, line index="输出信号波形 2") -> (output string=w913:string)
            n501 = VISA Write(VISA resource name=w917, write buffer=w913, error in (no error)=w910) -> (VISA resource name out=w912:refnum<visa-resource-name>, error out=w911:errorcluster)  [unwired: 1 out]
          }
          frame #1 {
            n502 = Wait (ms)(milliseconds to wait=u32 150) -> ()  [unwired: 1 out]
          }
          frame #2 {
            n503 = Number To Fractional String(use system decimal point (T)=TRUE ("使用系统小数点(T)"), number="低电平/V 2") -> (F-format string=w921:string)  [unwired: 2 in]
            n504 = Concatenate Strings ("连接字符串")(w923, ":VOLTage:LOW ", w921) -> (w920:string)
            n505 = VISA Write(VISA resource name=w927, write buffer=w920, error in (no error)=w926) -> (VISA resource name out=w925:refnum<visa-resource-name>, error out=w924:errorcluster)  [unwired: 1 out]
          }
          frame #3 {
            n506 = Wait (ms)(milliseconds to wait=u32 150) -> ()  [unwired: 1 out]
          }
          frame #4 {
            # "1 频率"
            n507 = Concatenate Strings(w930, ":FREQ ") -> (w937:string)
            n508 = Format Into String ("格式化写入字符串")(initial string=w937, "频率/Hz 2") -> (resulting string=w938:string)  [unwired: 2 in, 1 out]
            n509 = VISA Write(VISA resource name=w936, write buffer=w938, error in (no error)=w935) -> (VISA resource name out=w934:refnum<visa-resource-name>, error out=w931:errorcluster)  [unwired: 1 out]
          }
          frame #5 {
            n510 = Wait (ms)(milliseconds to wait=u32 150) -> ()  [unwired: 1 out]
          }
          frame #6 {
            n511 = Number To Fractional String(use system decimal point (T)=TRUE ("使用系统小数点(T)"), number="高电平/V 2") -> (F-format string=w943:string)  [unwired: 2 in]
            n512 = Concatenate Strings(w946, ":VOLTage:HIGH ", w943) -> (w945:string)
            n513 = VISA Write(VISA resource name=w942, write buffer=w945, error in (no error)=w941) -> (VISA resource name out=w949:refnum<visa-resource-name>, error out=w948:errorcluster)  [unwired: 1 out]
          }
          frame #7 {
            n514 = Wait (ms)(milliseconds to wait=u32 150) -> ()  [unwired: 1 out]
          }
          frame #8 {
            n515 = Pick Line(multi-line string=":OUTP1:IMPedance \n:OUTP2:IMPedance " ("write buffer"), line index=w951) -> (output string=w955:string)  [unwired: 1 in]
            n516 = Concatenate Strings ("连接字符串")(w957, w955, "INFINITY") -> (w958:string)
            n517 = VISA Write(VISA resource name=w960, write buffer=w958, error in (no error)=w959) -> (VISA resource name out=w954:refnum<visa-resource-name>, error out=w953:errorcluster)  [unwired: 1 out]
          }
          frame #9 {
            n518 = Wait (ms)(milliseconds to wait=u32 150) -> ()  [unwired: 1 out]
          }
          frame #10 {
            n519 = Number To Fractional String(use system decimal point (T)=TRUE ("使用系统小数点(T)"), number="占空比/% 2") -> (F-format string=w969:string)  [unwired: 2 in]
            n520 = Concatenate Strings(w967, ":PULSe:DCYCle ", w969) -> (w964:string)
            n521 = VISA Write(VISA resource name=w966, write buffer=w964, error in (no error)=w965) -> (VISA resource name out=w962:refnum<visa-resource-name>, error out=w963:errorcluster)  [unwired: 1 out]
          }
          frame #11 {
            n522 = Wait (ms)(milliseconds to wait=u32 150) -> ()  [unwired: 1 out]
          }
          frame #12 {
            n523 = Number To Fractional String(use system decimal point (T)=TRUE ("使用系统小数点(T)"), number="延时/s 2") -> (F-format string=w980:string)  [unwired: 2 in]
            n524 = Concatenate Strings(w977, ":PULSe:DELay ", w980) -> (w978:string)
            n525 = VISA Write(VISA resource name=w976, write buffer=w978, error in (no error)=w975) -> (VISA resource name out=w974:refnum<visa-resource-name>, error out=w973:errorcluster)  [unwired: 1 out]
          }
          frame #13 {
            n526 = Wait (ms)(milliseconds to wait=u32 150) -> ()  [unwired: 1 out]
          }
          frame #14 {
            w992 = ":LEADing\n:TRAiling "  # Channel
            w996 = ":PULSe:TRANsition"  # VOLTage:Offset
            n527 = Pick Line(multi-line string=w992, line index="上升下降沿 2") -> (output string=w990:string)  [unwired: 1 in]
            n528 = Number To Fractional String(use system decimal point (T)=TRUE ("使用系统小数点(T)"), number="上升下降沿/s 2") -> (F-format string=w991:string)  [unwired: 2 in]
            n529 = Concatenate Strings(w984, w996, w990, w991) -> (w993:string)
            n530 = VISA Write(VISA resource name=w989, write buffer=w993, error in (no error)=w988) -> (VISA resource name out=w987:refnum<visa-resource-name>, error out=w986:errorcluster)  [unwired: 1 out]
          }
        }
        n531 = VISA Close(VISA resource name=w896, error in (no error)=w895) -> (error out=→"configure error out":errorcluster)
      }
    }
    n532 = event shown="[1] \"照明光\": 值改变" {
      selector: _ -> [_ _]
      dyn-events: _ -> [_ _]
      timeout: 0 -> [_ _]
      tunnel: "照明光" -> [_ w62]
      event Timeout {
        n533 = event-data() -> ()  [unwired: 1 in, 3 out]
      }
      event "照明光": Value Change {
        n534 = event-data() -> ()  [unwired: 1 in, 6 out]
        n535 = local read "stop bits (10: 1 bit)"() -> (w75:u16)
        n536 = local read "parity (0:none)"() -> (w74:enum16{"None", "Odd", "Even", "Mark", "Space"})
        n537 = local read "照明光VISA"() -> (w71:refnum<visa-resource-name>)
        n538 = local read "baud rate"() -> (w72:u32)
        n539 = local read "data bits (8)"() -> (w73:u16)
        n540 = call-poly "VISA Configure Serial Port"("VISA resource name"=w71, "baud rate (9600)"=w72, "data bits (8)"=w73, "parity (0:none)"=w74, "stop bits (10: 1 bit)"=w75) -> ("VISA resource name out"=w68:refnum<visa-resource-name>, "error out"=w67:errorcluster)  [unwired: 9 in]
        n541 = call <vilib>:"Simple Error Handler.vi"("error in (no error)"=w67) -> ()  [unwired: 4 in, 5 out]
        n542 = VISA Open(access mode=0, error in (no error)=w67, VISA resource name=w68) -> (VISA resource name=w70:refnum<visa-resource-name>, error out=w69:errorcluster)  [unwired: 2 in]
        n543 = stacked-sequence {
          tunnel: w70 -> [w80]
          tunnel: w69 -> [w79]
          tunnel: [w78] -> w65
          tunnel: [w77] -> w66
          tunnel: w62 -> [w76]
          frame #0 {
            n544 = case shown="假" w76 {
              tunnel: w80 -> [w86 w96]
              tunnel: [w84 w95] -> w78
              tunnel: w79 -> [w85 w94]
              tunnel: [w83 w93] -> w77
              frame False {
                n545 = Concatenate Strings(" \u0001\u0001¢", "\r") -> (w87:string)
                n546 = VISA Write(VISA resource name=w86, write buffer=w87, error in (no error)=w85) -> (VISA resource name out=w84:refnum<visa-resource-name>, error out=w83:errorcluster)  [unwired: 1 out]
                n547 = Wait (ms)(milliseconds to wait=50) -> ()  [unwired: 1 out]
              }
              frame True {
                w89 = " \u0001\u0000¡"  # Channel
                n548 = Wait (ms)(milliseconds to wait=50) -> ()  [unwired: 1 out]
                n549 = Concatenate Strings(w89, "\r") -> (w90:string)
                n550 = VISA Write(VISA resource name=w96, write buffer=w90, error in (no error)=w94) -> (VISA resource name out=w95:refnum<visa-resource-name>, error out=w93:errorcluster)  [unwired: 1 out]
              }
            }
          }
        }
        n551 = VISA Close(VISA resource name=w65, error in (no error)=w66) -> (error out=w64:errorcluster)
        n552 = call <vilib>:"Simple Error Handler.vi"("error in (no error)"=w64) -> ()  [unwired: 4 in, 5 out]
      }
    }
  }
  n553 = flat-sequence {
    frame #0 {
      "Backlight" <- i32[][] [] ("Backlight")
    }
    frame #1 {
      w1087 = FALSE
      # "删除背景光控件\n初始值设定"
      n554 = local write "cut backlight"(w1087) -> ()
      "backlight" <- w1087
    }
  }
  n555 = stacked-sequence {
    seq-local: [_ _ _ w1108 _ _ _ _] -> [_ _ _ _ w1126 w1146 w1149 w1351]
    seq-local: [_ _ _ w1107 _ _ _ _] -> [_ _ _ _ w1127 w1147 w1148 w1352]
    frame #0 {
      # "initialize all variables"
      n556 = property on="initialize" class="Bool"("Désactivé"=u8 0) -> ()  [unwired: 2 in, 2 out]
      n557 = property on="Acquire" class="Bool"("Visible"=FALSE) -> ()  [unwired: 2 in, 2 out]
      n558 = property on="Setup" class="Bool"("Visible"=FALSE) -> ()  [unwired: 2 in, 2 out]
      n559 = local write "indicator"("" ("indicator")) -> ()
      n560 = local write "initialized ?"(FALSE ("initialized ?")) -> ()
      n561 = local write "Continuous"(FALSE ("Continuous")) -> ()
      n562 = local write "Close"(FALSE ("Close")) -> ()
      n563 = property on="Device Name" class="Ring (严格)"("Désactivé"=u8 0) -> ()  [unwired: 2 in, 2 out]
      n564 = property on="Continuous" class="Bool (严格)"("Visible"=FALSE) -> ()  [unwired: 2 in, 2 out]
      n565 = local write "Commande tab"(T1."Settings" ("Commande tab")) -> ()
    }
    frame #1 {
      # "Read Uniq ID"
      n566 = stacked-sequence {
        frame #0 {
          n567 = call "read detector uniq-id.vi"() -> ("nbr of components"=w1100:i32, "UniqueID"=w1099:string[], "Name"=w1098:string[])  [unwired: 4 out]
          n568 = for {
            N: w1100 -> [_]
            tunnel: w1099 -> [w1102]
            tunnel: w1098 -> [w1101]
            n569 = property on="Device Name" class="Ring (严格)"("Chaînes []"=w1101) -> ()  [unwired: 2 in, 2 out]
            n570 = property on="Uniques ID" class="Ring (严格)"("Chaînes []"=w1102) -> ()  [unwired: 2 in, 2 out]
          }
        }
      }
    }
    frame #2 {
      n571 = while {
        stop <- "initialize" stop-if-true
        n572 = local read "Device Name"() -> (w1105:u16)
        n573 = local write "Uniques ID"(w1105) -> ()
        n574 = local read "Close"() -> (w1103:bool)
        n575 = Stop(stop? (T)=w1103) -> ()
        n576 = Wait Until Next ms Multiple(millisecond multiple=u32 100 ("n millisecondes")) -> ()  [unwired: 1 out]
      }
    }
    frame #3 {
      n577 = stacked-sequence {
        tunnel: [_ w1115 _ _] -> w1108
        tunnel: [_ w1114 _ _] -> w1107
        frame #0 {
          n578 = local write "indicator"("Initializing ..." ("indicator")) -> ()
        }
        frame #1 {
          n579 = local read "Uniques ID"() -> (w1112:u16)
          n580 = property on="Uniques ID" class="Ring (严格)"() -> ("Chaînes []"=w1113:string[])  [unwired: 2 in, 2 out]
          n581 = Index Array(array=w1113, index=w1112) -> (element=w1111:string)
          n582 = call "Initialize CCD.vi"("Unique id:"=w1111) -> ("activeYPixels"=→"Y Pixels:":i32, "JYCCDLib.IJYCCDReqd"=w1114:refnum<k7>, "activeXPixels"=→"X Pixels:":i32, "sortie d'erreur"=w1115:errorcluster, "FirmwareVersion"=→"Firmware\nVersion":string)  [unwired: 3 out]
        }
        frame #2 {
          n583 = property on="initialize" class="Bool"("Désactivé"=u8 2) -> ()  [unwired: 2 in, 2 out]
          n584 = property on="Device Name" class="Ring (严格)"("Désactivé"=u8 2) -> ()  [unwired: 2 in, 2 out]
          n585 = local write "Continuous"(FALSE ("Continuous")) -> ()
          n586 = property on="Setup" class="Bool"("Visible"=TRUE) -> ()  [unwired: 2 in, 2 out]
        }
        frame #3 {
          n587 = local write "initialized ?"(TRUE ("initialized ?")) -> ()
          n588 = local write "indicator"("Initialized !" ("indicator")) -> ()
        }
      }
    }
    frame #4 {
      # "Actually not working"
      # "Read ADC and GAIN"
      n589 = case shown="真" "Constante de condition\n(Voir l'aide contextuelle)" {
        tunnel: w1127 -> [_ w1137]
        tunnel: w1126 -> [_ w1136]
        frame False {
        }
        frame True {
          # "Read Input supported trigger"
          n590 = call "Trigger - Get Supported Input.vi"("JYCCDLib.IJYCCDReqd"=w1137, "Error Input"=w1136) -> ("trigAddress"=w1131:i32, "eventPtr"=w1132:i32, "trigEventString"=w1135:string, "trigSigType"=w1134:i32, "trigSigTypeString"=w1133:string)  [unwired: 4 out]
          n591 = local write "trigSigTypeString"(w1133) -> ()
          n592 = local write "trigAddress"(w1131) -> ()
          n593 = local write "Trigger Type :"(w1132) -> ()
          n594 = local write "trigEventString"(w1135) -> ()
          n595 = local write "Signal type :"(w1134) -> ()
        }
      }
      n596 = call "Init ADC & Gain.vi"("JYCCDLib.IJYCCDReqd"=w1127, "input error"=w1126) -> ("ADC Number"=w1125:i32[], "ADC description"=w1130:string[], "Gain Number"=w1128:i32[], "Gain description"=w1129:string[])
      n597 = local write "Gain Number"(w1128) -> ()
      n598 = local write "ADC Number"(w1125) -> ()
      n599 = stacked-sequence {
        tunnel: w1130 -> [w1138 _]
        tunnel: w1129 -> [_ w1139]
        frame #0 {
          n600 = property on="ADC" class="Ring (严格)"("Chaînes []"=w1138) -> ()  [unwired: 2 in, 2 out]
        }
        frame #1 {
          n601 = property on="GAIN" class="Ring (严格)"("Chaînes []"=w1139) -> ()  [unwired: 2 in, 2 out]
        }
      }
    }
    frame #5 {
      # "IS multi Accumulation Supported ?"
      n602 = call "MultiAccu - Is Supported.vi"("Error In"=w1146, "JYCCDLib.IJYCCDReqd"=w1147) -> ("IsOperatingModeSupported"=w1140:bool)  [unwired: 3 out]
      n603 = Select(t=0, s=w1140, f=2) -> (s? t:f=w1143:i32)
      n604 = Select(t=FALSE, s=w1140, f=w1140) -> (s? t:f=w1142:bool)
      n605 = local write "Multi Accumulation mode:"(w1142) -> ()
      n606 = property on="Multi Accumulation mode:" class="Bool (严格)"("Désactivé"=w1143) -> ()  [unwired: 2 in, 2 out]
      n607 = property on="Multi Accumulation mode:" class="Bool (严格)"("Désactivé"=w1143) -> ()  [unwired: 2 in, 2 out]
    }
    frame #6 {
      n608 = while {
        tunnel: w1148 -> [w1156]
        tunnel: w1149 -> [w1155]
        stop <- "Close" stop-if-true
        n609 = local read "Continuous"() -> (w1157:bool)
        n610 = case shown="假" "Reformat" {
          frame False {
          }
          frame True {
            n611 = local read "Y Pixels:"() -> (w1329:i32)
            n612 = local read "X Pixels:"() -> (w1331:i32)
            n613 = call "Spectral Reformat CCD area.vi"("Y Pixels:"=w1329, "X Pixels:"=w1331, "numAreas"="Number of Areas :") -> ("areas :"=→"areas :":i32[][])  [unwired: 3 out]
          }
        }
        n614 = local read "Accumulations:"() -> (w1152:u16)
        n615 = Or(x="Acquire", y=w1157) -> (x .or. y?=w1154:bool)
        n616 = case shown="真" w1154 {
          tunnel: w1156 -> [_ w1169]
          tunnel: w1155 -> [_ w1168]
          tunnel: "Enable InputTriggers :" -> [_ w1167]
          tunnel: "Multi Accumulation mode:" -> [_ w1166]
          tunnel: w1152 -> [_ w1165]
          tunnel: "MultiAcqShutterMode" -> [_ w1164]
          frame False {
          }
          frame True {
            n617 = stacked-sequence {
              seq-local: [_ _ w1182 _ _] -> [_ _ _ w1255 _]
              seq-local: [_ _ _ w1228 _] -> [_ _ _ _ w1295]
              tunnel: w1169 -> [_ w1171 w1186 w1254 _]
              tunnel: w1168 -> [_ w1172 w1185 w1253 _]
              tunnel: w1167 -> [_ w1173 _ _ _]
              tunnel: w1166 -> [_ _ w1184 _ _]
              tunnel: w1165 -> [_ _ w1183 _ _]
              tunnel: w1164 -> [_ _ w1181 _ _]
              frame #0 {
                n618 = local write "CCD Busy"(TRUE ("CCD Busy")) -> ()
              }
              frame #1 {
                n619 = case shown="真" w1173 {
                  tunnel: w1172 -> [w1174 w1180]
                  tunnel: w1171 -> [w1175 w1179]
                  frame False {
                    n620 = call "Trigger - Disable.vi"("Error In"=w1174, "JYCCDLib.IJYCCDReqd"=w1175) -> ()  [unwired: 6 out]
                  }
                  frame True {
                    n621 = local read "Trigger Type :"() -> (w1176:u16)
                    n622 = local read "Signal type :"() -> (w1177:enum16{"TTL Rising Edge", "TTL Falling Edge"})
                    n623 = local read "trigAddress"() -> (w1178:i32)
                    n624 = call "Trigger - Enable.vi"("Error In"=w1180, "sigType"=w1177, "event"=w1176, "trigAddress"=w1178, "JYCCDLib.IJYCCDReqd"=w1179) -> ()  [unwired: 3 out]
                  }
                }
              }
              frame #2 {
                n625 = case shown="真" w1184 {
                  selector: w1184 -> [_ w1215]
                  tunnel: w1186 -> [w1212 w1218]
                  tunnel: w1185 -> [w1211 w1217]
                  tunnel: w1183 -> [_ w1216]
                  tunnel: [u16 1 ("Accumulations:") w1216] -> w1182
                  tunnel: w1181 -> [_ w1214]
                  frame False {
                    n626 = call "MultiAccu - Disable.vi"("Error In"=w1211, "JYCCDLib.IJYCCDReqd"=w1212) -> ()  [unwired: 4 out]
                  }
                  frame True {
                    n627 = call "MultiAccu - Configure.vi"("JYCCDLib.IJYCCDReqd"=w1218, "Cleans Before"="Number of Cleans", "Accumulations:"=w1216, "MultiAcqHardwareMode"=w1215, "MultiAcqShutterMode"=w1214, "Error In"=w1217) -> ()  [unwired: 1 in, 9 out]
                  }
                }
                n628 = flat-sequence {
                  frame #0 {
                    n629 = Current VI's Path() -> (path=w1192:path)
                    n630 = Get Date/Time In Seconds() -> (seconds since 1Jan1904=w1194:timestamp)
                    n631 = Strip Path(path=w1192) -> (stripped path=w1193:path)  [unwired: 1 out]
                    n632 = Path To String(path=w1193) -> (string=w1195:string)
                    n633 = Format Date/Time String(time format string (%c)="%m.%d" ("时间格式字符串(%c)"), seconds (now)=w1194) -> (date/time string=w1201:string)  [unwired: 1 in]
                    n634 = Concatenate Strings(w1195, "\\Save\\" ("字符串"), w1201) -> (w1196:string)
                    n635 = String To Path(string=w1196) -> (path=w1197:path)
                    n636 = call <vilib>:"Check if File or Folder Exists.vi"("path"=w1197) -> ("file or folder exists?"=w1198:bool, "dup path"=w1200:path)  [unwired: 8 in, 1 out]
                    n637 = case shown="真" w1198 {
                      tunnel: [w1208 w1209] -> w1199
                      tunnel: w1200 -> [w1207 w1209]
                      tunnel: w1201 -> [w1206 _]
                      frame False {
                        n638 = Create Folder(prompt (Create Folder)=w1206, path (use dialog)=w1207) -> (created path=w1208:path)  [unwired: 1 in, 2 out]
                      }
                      frame True {
                      }
                    }
                    n639 = Format Date/Time String(time format string (%c)="%y%m%d%H%M%S " ("时间格式字符串(%c)"), seconds (now)=w1194) -> (date/time string=w1204:string)  [unwired: 1 in]
                    n640 = Path To String(path=w1199) -> (string=w1202:string)
                    n641 = Concatenate Strings(w1202, "\\" ("字符串")) -> (w1203:string)
                    n642 = Concatenate Strings(w1203, w1204) -> (w1191:string)
                    n643 = String To Path(string=w1191) -> (path=→"最终存储路径 2":path)
                  }
                }
              }
              frame #3 {
                n644 = local read "cut backlight"() -> (w1242:bool)
                n645 = local read "backlight"() -> (w1241:bool)
                n646 = call "MultiAccu - Acquire spectral.vi"("error in"=w1253, "Accumulations:"=w1255, "ShutterOpen"="ShutterOpen", "JYCCDLib.IJYCCDReqd"=w1254) -> ("Acq Time(ms)"=→"Acq Time(ms)":u32, "Array Out"=w1252:i32[][][])  [unwired: 1 out]
                n647 = And(x=w1242, y=w1241) -> (x .and. y?=w1243:bool)
                n648 = call "Array reset dimension.vi"("Area Number"="Area Number to Display", "Array In"=w1252) -> ("Array Out"=w1244:i32[][])
                n649 = case shown="真" w1243 {
                  tunnel: [w1291 w1292] -> w1245
                  tunnel: w1244 -> [w1291 w1293]
                  frame False {
                  }
                  frame True {
                    n650 = local read "Backlight"() -> (w1294:i32[][])
                    n651 = Subtract(x=w1293, y=w1294) -> (x-y=w1292:i32[][])
                  }
                }
                n652 = local read "波长范围"() -> (w1220:dbl[])
                n653 = local write "Data"(w1244) -> ()
                n654 = Index Array(array=w1245, index (row)=0 ("禁用的索引 (列)")) -> (element=w1246:i32[])  [unwired: 1 in]
                n655 = Reverse 1D Array(array=w1246) -> (reversed array=w1229:i32[])
                n656 = call "转换至动态数据2"("Array"=w1220) -> ("Dynamic Data Type"=w1248:dynamicdata)  [unwired: 3 in]
                n657 = call "转换至动态数据"("Array"=w1229) -> ("Dynamic Data Type"=w1249:dynamicdata)  [unwired: 3 in]
                n658 = call <vilib>:"Median Filter.vi"("left rank"=6, "X"=w1229) -> ("Filtered X"=w1234:dbl[])  [unwired: 8 in, 1 out]
                n659 = call "Build XY Graph2"("Y Input"=w1249, "X Input"=w1248) -> ("XY Graph"=w1247:cluster{"Y":dbl[], "Y":dbl[]}[])  [unwired: 8 in, 1 out]
                n660 = Subtract(x="拟合终点", y="拟合起点") -> (x-y=w1223:i32)
                n661 = local write "Spectrum"(w1247) -> ()
                n662 = local read "滤波阈值"() -> (w1238:dbl)
                n663 = Array Subset(array=w1220, index="拟合起点", length=w1223) -> (w1226:dbl[])
                n664 = local read "拟合参数"() -> (w1219:dbl[])
                n665 = In Range and Coerce(upper limit=w1238, x=w1234, lower limit=-100.0) -> (In Range?=w1237:bool[])  [unwired: 1 out]
                n666 = Not(x=w1237) -> (.not. x?=w1231:bool[])
                n667 = local read "滤波阈值"() -> (w1233:dbl)
                n668 = local write "范围内？"(w1237) -> ()
                n669 = local read "X Pixels:"() -> (w1235:i32)
                n670 = Or Array Elements(Boolean array=w1231) -> (logical OR=w1236:bool)
                n671 = case shown="真" w1236 {
                  tunnel: w1235 -> [_ w1278]
                  tunnel: w1234 -> [w1274 w1277]
                  tunnel: [w1274 w1276] -> w1222
                  tunnel: w1233 -> [_ w1275]
                  frame False {
                  }
                  frame True {
                    n672 = for {
                      N: w1278 -> [_]
                      tunnel: w1277 -> [w1282] mode=indexing
                      tunnel: [w1281] -> w1276 mode=indexing
                      shift-right: [w1281] -> _
                      shift-left: _ -> [w1280]
                      tunnel: w1275 -> [w1279]
                      n673 = Greater?(x=w1282, y=w1279) -> (0:w1284:bool)
                      n674 = Less?(x=w1282, y=-100.0) -> (x < y?=w1285:bool)
                      n675 = Or(x=w1284, y=w1285) -> (x .or. y?=w1283:bool)
                      n676 = case shown="真" w1283 {
                        tunnel: w1282 -> [w1287 _]
                        tunnel: [w1287 w1289] -> w1281
                        tunnel: w1280 -> [_ w1290]
                        frame False {
                        }
                        frame True {
                          n677 = call <vilib>:"Median Filter PtByPt.vi"("rank"=5, "x"=w1290) -> ("Filtered x"=w1289:dbl)  [unwired: 2 in, 1 out]
                        }
                      }
                    }
                  }
                }
                n678 = Array Subset(array=w1222, index="拟合起点", length=w1223) -> (w1225:dbl[])
                n679 = Bundle("波长范围"=w1220, "Filtered X"=w1222) -> (w1221:cluster{"波长范围 ":dbl[], "Filtered X":dbl[]})  [unwired: 1 in]
                n680 = case shown="真" "是否拟合" {
                  tunnel: w1225 -> [w1258 w1264]
                  tunnel: w1226 -> [_ w1263]
                  tunnel: [w1258 w1262] -> w1240
                  tunnel: w1221 -> [_ w1260]
                  frame False {
                  }
                  frame True {
                    n681 = call "转换至动态数据7"("Array"=w1264) -> ("Dynamic Data Type"=w1269:dynamicdata)  [unwired: 3 in]
                    n682 = call "转换至动态数据8"("Array"=w1263) -> ("Dynamic Data Type"=w1270:dynamicdata)  [unwired: 3 in]
                    n683 = call "曲线拟合2"("Locations"=w1270, "Signals"=w1269) -> ("best fit"=w1267:dynamicdata, "non-linear coefficients"=w1268:dynamicdata)  [unwired: 5 in, 3 out]
                    n684 = call "从动态数据转换3"("Dynamic Data Type"=w1268) -> ("Array"=w1271:dbl[])  [unwired: 3 in]
                    n685 = call "从动态数据转换4"("Dynamic Data Type"=w1267) -> ("Array"=w1262:dbl[])  [unwired: 3 in]
                    n686 = Index Array(array=w1271, index #1=0 ("索引"), index #2=1 ("索引")) -> (element #1=w1273:dbl, element #2=w1272:dbl)
                    n687 = local write "拟合参数"(w1271) -> ()
                    n688 = local write "xc"(w1273) -> ()
                    n689 = Bundle(w1263, "Array"=w1262) -> (w1261:cluster{dbl[], "Array":dbl[]})  [unwired: 1 in]
                    n690 = local write "w"(w1272) -> ()
                    n691 = Build Array(w1260, w1261) -> (→"best fit":cluster{"波长范围 ":dbl[], "Array":dbl[]}[])
                  }
                }
                n692 = Build Array(w1226, w1229, w1240, w1219) -> (w1228:dbl[][])
              }
              frame #4 {
                n693 = case shown="真" "是否保存" {
                  tunnel: w1295 -> [_ w1299]
                  frame False {
                  }
                  frame True {
                    n694 = Get Date/Time In Seconds() -> (seconds since 1Jan1904=w1313:timestamp)
                    n695 = Get Date/Time String(date format (0)=enum16{"short", "long", "abbreviated"}."abbreviated" ("日期格式(0)"), seconds (now)=w1313, want seconds? (F)=TRUE ("需要秒？(F)")) -> (date string=w1311:string, time string=w1312:string)
                    n696 = Search and Replace String(replace all?=TRUE ("替换全部？(F)"), input string=w1312, search string=":" ("搜索字符串"), replace string="-" ("替换字符串(\"\")")) -> (result string=w1310:string)  [unwired: 4 in, 3 out]
                    n697 = local read "最终存储路径 2"() -> (w1314:path)
                    n698 = Path To String(path=w1314) -> (string=w1317:string)
                    n699 = Concatenate Strings(w1317, w1311, w1310, "光谱" ("字符串"), ".xls" ("字符串")) -> (w1316:string)
                    n700 = String To Path(string=w1316) -> (path=w1315:path)
                    n701 = call-poly <vilib>:"Write Delimited Spreadsheet.vi"("file path (dialog if empty)"=w1315, "format (%.3f)"="%.16f", "2D data"=w1299, "append to file? (new file:F)"=TRUE ("append to file? (F)"), "transpose? (no:F)"=TRUE ("transpose? (F)")) -> ()  [unwired: 9 in, 2 out]
                  }
                }
                n702 = case shown="真" "Save Backlight" {
                  frame False {
                  }
                  frame True {
                    w1318 = TRUE ("删除背景光")
                    n703 = local read "Data"() -> (w1320:i32[][])
                    n704 = local write "Backlight"(w1320) -> ()
                    n705 = local write "cut backlight"(w1318) -> ()
                    n706 = local write "backlight"(w1318) -> ()
                    n707 = local write "Save Backlight"(FALSE ("Save Backlight")) -> ()
                  }
                }
                n708 = local write "CCD Busy"(FALSE ("CCD Busy")) -> ()
              }
            }
          }
        }
        n709 = case shown="假" "Setup" {
          tunnel: w1155 -> [_ w1334]
          tunnel: w1156 -> [_ w1333]
          frame False {
          }
          frame True {
            n710 = stacked-sequence {
              tunnel: w1334 -> [_ w1348 _]
              tunnel: w1333 -> [_ w1336 _]
              frame #0 {
                n711 = local write "indicator"("Setting up the detector" ("indicator")) -> ()
              }
              frame #1 {
                w1346 = 1 items=["JYMCD_ACQ_FORMAT_IMAGE", "JYMCD_ACQ_FORMAT_SCAN"] ("Acquisition type")
                n712 = local read "Gain Number"() -> (w1341:i32[])
                n713 = local read "GAIN"() -> (w1337:u16)
                n714 = local read "ADC Number"() -> (w1342:i32[])
                n715 = local read "ADC"() -> (w1338:u16)
                n716 = Index Array(array=w1341, index=w1337) -> (element=w1339:i32)
                n717 = Index Array(array=w1342, index=w1338) -> (element=w1340:i32)
                n718 = local read "Number of Areas :"() -> (w1344:u16)
                n719 = local read "areas :"() -> (w1345:i32[][])
                n720 = call "Setup CCD.vi"("numAreas"=w1344, "areas :"=w1345, "JYCCDLib.IJYCCDReqd"=w1336, "entrée d'erreur (pas d'erreur)"=w1348, "Acquisition type"=w1346, "Gain"=w1339, "Select ADC"=w1340, "Integration time(ms)"="Integration time (ms) :") -> ("DataSize"=→"DataSize":i32)  [unwired: 1 out]
                "JYCCDLib.IJYCCDReqd" <- w1336
              }
              frame #2 {
                w1349 = TRUE ("Visible")
                n721 = property on="Continuous" class="Bool (严格)"("Visible"=w1349) -> ()  [unwired: 2 in, 2 out]
                n722 = property on="Acquire" class="Bool"("Visible"=w1349) -> ()  [unwired: 2 in, 2 out]
                n723 = local write "indicator"("Ready !" ("indicator")) -> ()
              }
            }
          }
        }
        n724 = case shown="假" "Temperature" {
          tunnel: w1156 -> [_ w1323]
          tunnel: w1155 -> [_ w1322]
          frame False {
            n725 = property on="temp graph" class="WFChart (严格)"("Visible"=FALSE) -> ()  [unwired: 2 in, 2 out]
          }
          frame True {
            n726 = stacked-sequence {
              tunnel: w1323 -> [_ w1328]
              tunnel: w1322 -> [_ w1327]
              frame #0 {
                n727 = property on="temp graph" class="WFChart (严格)"("Visible"=TRUE) -> ()  [unwired: 2 in, 2 out]
              }
              frame #1 {
                w1326 = u16 0 items=["° Celsius", "Kelvin", "° Farenheit"] ("units")
                n728 = call "read temperature.vi"("entrée d'erreur (pas d'erreur)"=w1327, "units"=w1326, "JYCCDLib.IJYCCDReqd"=w1328) -> ("Current Temperature"=w1325:dbl)
                n729 = local write "temp graph"(w1325) -> ()
              }
            }
          }
        }
        n730 = Wait Until Next ms Multiple(millisecond multiple=u32 50 ("n millisecondes")) -> ()  [unwired: 1 out]
      }
    }
    frame #7 {
      n731 = Close Reference(reference=w1352, error in (no error)=w1351) -> ()  [unwired: 1 out]
    }
  }
  n732 = stacked-sequence {
    seq-local: [_ _ w1362 _ _] -> [_ _ _ w1372 w1377]
    seq-local: [_ _ w1361 _ _] -> [_ _ _ w1371 _]
    seq-local: [_ _ _ w1370 _] -> [_ _ _ _ _]
    frame #0 {
      n733 = call "Get Monos From Config Browser.vi"() -> ("UniqueIDs"=w1357:string[], "Mono ID"=w1358:string[])  [unwired: 3 in, 1 out]
      n734 = Build Cluster Array(w1358, w1357) -> (w1355:cluster{"String":string, "String":string}[])
      n735 = property on="Mono ID" class="CmbBox"("Strings And Values []"=w1355) -> ()  [unwired: 2 in, 2 out]
      n736 = Index Array(array=w1355, index=0) -> (element=w1356:cluster{"String":string, "String":string})
      n737 = Unbundle(w1356) -> ("String"=w1353:string)  [unwired: 1 out]
      "Current UniqueID" <- w1353
      n738 = local write "Mono ID"(w1353) -> ()
    }
    frame #1 {
      n739 = while {
        stop <- "Connect" stop-if-true
        n740 = local read "Mono ID"() -> (w1359:string)
        n741 = local write "Current UniqueID"(w1359) -> ()
      }
    }
    frame #2 {
      n742 = local read "Mono ID"() -> (w1364:string)
      n743 = call "JYInitMono.vi"("Unique ID"=w1364, "Force Init"="Force\nInitialization") -> ("Refnum out"=w1362:refnum<k7>, "Initialized"=→"Initialized JY":bool, "error out"=w1361:errorcluster)  [unwired: 9 in, 2 out]
    }
    frame #3 {
      n744 = call "Show Current Grating.vi"("Refnum in"=w1372, "error in (no error)"=w1371) -> ("Gratings"=w1373:dbl[], "Grating Index"=w1367:i32, "Current Grating"=w1369:dbl, "Current Description"=w1366:string, "error out"=w1370:errorcluster)  [unwired: 5 in, 4 out]
      "Gratings" <- w1373
      n745 = local write "Current Grating"(w1369) -> ()
      n746 = local write "Current Description"(w1366) -> ()
      n747 = Number To Decimal String(number=w1373) -> (decimal integer string=w1375:string[])  [unwired: 1 in]
      n748 = Number To Decimal String(number=w1367) -> (decimal integer string=w1368:string)  [unwired: 1 in]
      n749 = property on="Target Grating" class="CmbBox"("Value"=w1368) -> ()  [unwired: 2 in, 2 out]
      n750 = Build Cluster Array(w1375, string[] ["1", "2", "3"]) -> (w1376:cluster{"Numeric":string, string}[])
      n751 = property on="Target Grating" class="CmbBox"("Strings And Values []"=w1376) -> ()  [unwired: 2 in, 2 out]
    }
    frame #4 {
      n752 = while {
        tunnel: w1377 -> [w1379]
        stop <- w1378 stop-if-true
        n753 = stacked-sequence {
          seq-local: [w1383 _ _ _ _] -> [_ w1390 w1401 _ w1409]
          seq-local: [w1382 _ _ _ _] -> [_ w1389 w1400 _ _]
          seq-local: [_ w1388 _ _ _] -> [_ _ _ _ _]
          seq-local: [_ w1387 _ _ _] -> [_ _ _ _ _]
          seq-local: [_ _ w1393 _ _] -> [_ _ _ _ _]
          seq-local: [_ _ w1392 _ _] -> [_ _ _ w1403 _]
          tunnel: w1379 -> [w1381 _ _ w1404 _]
          frame #0 {
            n754 = call "Show Current Grating.vi"("Refnum in"=w1381) -> ("Grating Index"=→"Grating Index":i32, "Current Grating"=→"Current Grating":dbl, "Current Description"=→"Current Description":string, "error out"=w1382:errorcluster, "JYMONOLib.IJYMonoReqd"=w1383:refnum<k7>)  [unwired: 6 in, 4 out]
          }
          frame #1 {
            n755 = call "JYGetCurrentWL.vi"("error in (no error)"=w1389, "JYMONOLib.IJYMonoReqd"=w1390) -> ("error out"=w1387:errorcluster, "Units"=→"Units":string, "Current WL"=→"Current WL":dbl, "JYMONOLib.IJYMonoReqd 2"=w1388:refnum<k7>)  [unwired: 6 in]
          }
          frame #2 {
            w1398 = u16 1 items=["Entrance", "Exit"] ("Mirror Number")
            w1399 = u16 0 items=["Entrance", "Exit"] ("Mirror Number")
            n756 = call "JYGetMirrorPos.vi"("error in (no error)"=w1400, "Mirror"=w1399, "Refnum In"=w1401) -> ("error out"=w1396:errorcluster, "Current Mirror Position"=→"Entrance Mirror\nPosition":i32, "Refnum Out"=w1397:refnum<k7>)  [unwired: 1 in]
            n757 = call "JYGetMirrorPos.vi"("error in (no error)"=w1396, "Mirror"=w1398, "Refnum In"=w1397) -> ("error out"=w1392:errorcluster, "Current Mirror Position"=→"Exit Mirror\nPosition":i32, "Refnum Out"=w1393:refnum<k7>)  [unwired: 1 in]
          }
          frame #3 {
            w1406 = u16 0 items=["Front Entrance", "Side Entrance", "Front Exit", "Side Exit", "First Intermediate", "Second Intermediate"] ("Slit")
            n758 = call "JYGetSlits.vi"("MonoRefNum IN"=w1404, "Slit"=w1406, "error in (no error)"=w1403) -> ("Units"=→"Units 2":string, "Slit Width"=→"Front Entrance":dbl, "error out"=→"error out":errorcluster)  [unwired: 13 in, 1 out]
          }
          frame #4 {
            n759 = case shown="假" "Move To\nTarget Positions" {
              tunnel: w1409 -> [_ w1410]
              frame False {
              }
              frame True {
                n760 = stacked-sequence {
                  seq-local: [w1412 _ _ _] -> [_ w1418 _ _]
                  seq-local: [_ w1416 _ _] -> [_ _ w1433 _]
                  seq-local: [_ _ w1420 _] -> [_ _ _ w1439]
                  seq-local: [_ _ _ w1436] -> [_ _ _ _]
                  tunnel: w1410 -> [w1414 w1417 w1431 w1440]
                  frame #0 {
                    n761 = property on="Target Grating" class="CmbBox"() -> ("Value"=w1411:string)  [unwired: 2 in, 2 out]
                    n762 = local read "error out"() -> (w1413:errorcluster)
                    n763 = Decimal String To Number(string=w1411) -> (number=w1415:i32)  [unwired: 2 in, 1 out]
                    n764 = call "JYTurret.vi"("error in (no error)"=w1413, "Grating Index"=w1415, "JYMONOLib.IJYMonoReqd"=w1414) -> ("error out"=w1412:errorcluster)  [unwired: 2 out]
                  }
                  frame #1 {
                    # "Move Grating to Target Position"
                    n765 = call "JYMoveToWavelength.vi"("error in (no error)"=w1418, "Target WL"="Target WL", "RefNum In"=w1417) -> ("error out"=w1416:errorcluster)  [unwired: 1 in, 2 out]
                  }
                  frame #2 {
                    w1426 = u16 1 items=["Entrance", "Exit"] ("Mirror Number")
                    w1425 = u16 0 items=["Entrance", "Exit"] ("Mirror Number")
                    w1432 = u16 1 items=["Entrance", "Exit", "Front", "Side"] ("Mirror Number")
                    w1435 = u16 0 items=["Entrance", "Exit", "Front", "Side"] ("Mirror Number")
                    # "Move Mirrors"
                    n766 = call "JYMirrorMove.vi"("error in (no error)"=w1433, "Mirror Position"="Entrance Mirror", "Mirror Number"=w1435, "RefNum In"=w1431) -> ("error out"=w1430:errorcluster)  [unwired: 6 in, 1 out]
                    n767 = call "JYMirrorMove.vi"("error in (no error)"=w1430, "Mirror Position"="Exit Mirror", "Mirror Number"=w1432, "RefNum In"=w1431) -> ("error out"=w1423:errorcluster, "MonoRefNum Out"=w1424:refnum<k7>)  [unwired: 6 in]
                    n768 = call "JYGetMirrorPos.vi"("error in (no error)"=w1423, "Mirror"=w1425, "Refnum In"=w1424) -> ("error out"=w1428:errorcluster, "Current Mirror Position"=w1422:i32, "Refnum Out"=w1427:refnum<k7>)  [unwired: 1 in]
                    n769 = local write "Entrance Mirror\nPosition"(w1422) -> ()
                    n770 = call "JYGetMirrorPos.vi"("error in (no error)"=w1428, "Mirror"=w1426, "Refnum In"=w1427) -> ("error out"=w1420:errorcluster, "Current Mirror Position"=w1421:i32)  [unwired: 1 in, 1 out]
                    n771 = local write "Exit Mirror\nPosition"(w1421) -> ()
                  }
                  frame #3 {
                    w1438 = u16 0 items=["Front Entrance", "Side Entrance", "Front Exit", "Side Exit", "First Intermediate", "Second Intermediate"] ("Slit")
                    # "Set New Slit Positions"
                    n772 = call "JYSlits.vi"("JYMONOLib.IJYMonoReqd"=w1440, "Slit"=w1438, "error in (no error)"=w1439, "Slit Width"="Target\nFront Entrance") -> ("error out"=w1436:errorcluster)  [unwired: 1 in, 1 out]
                  }
                }
              }
            }
          }
        }
        n773 = local read "Close"() -> (w1378:bool)
      }
    }
  }
  n774 = flat-sequence {
    frame #0 {
      n775 = call <vilib>:"Create Report.vi"("window state (normal)"=T3."no change", "report type"=Report_Type."Excel", "template (empty)"=path "D:/desktop/train/TEST1/Save/516中心波长.xlsx") -> ("report out"=w1447:refnum<class "NI_report.lvclass">, "error out"=w1446:errorcluster)  [unwired: 11 in]
      n776 = call-poly <vilib>:"Excel Get Data.vi"("report in"=w1447, "data type"=string[][] [], "error in (no error)"=w1446) -> ("report out"=w1442:refnum<class "NI_report.lvclass">, "data"=w1450:string[][], "error out"=w1441:errorcluster)  [unwired: 10 in]
      n777 = call-dynamic "Dispose Report.vi"("report in"=w1442, "error in (no error)"=w1441) -> ()  [unwired: 13 in, 1 out]
      n778 = Index Array(array=w1450, index (col)=0 ("禁用的索引 (列)")) -> (element=w1452:string[])  [unwired: 1 in]
      n779 = Fract/Exp String To Number(string=w1452) -> (number=→"波长范围":dbl[])  [unwired: 3 in, 1 out]
    }
  }
